vi "SEC code V4.1.vi"() -> ()   [LabVIEW 2020]
uses:
  SEC code V3.1/Drivers and Aux files/user.lib/atmcd32d.llb/Shutter_type typedef.ctl
  SEC code V3.1/Drivers and Aux files/State.ctl
  SEC code V3.1/Drivers and Aux files/SECenumctl.ctl
  SEC code V3.1/Drivers and Aux files/user.lib/atmcd32d.llb/TriggerMode_mode typedef.ctl
  SEC code V3.1/Drivers and Aux files/OSSPEC.ctl
  SEC code V3.1/Drivers and Aux files/OSPEC-enum.ctl
  Labview/IVIUM/IVIUM_remdriver.lvlib
panel:
  in  "Tab Control 5":enum32{"IVIUM", "iDUS", "Kymera"}(tab)
  out "current":dbl caption="Current (A)" format="%_4g"
  out "cell on":bool
  out "V (during measurment)":dbl
  out "Potentiostat Status":string
  out "T reached?":bool
  out "Shut down sequence run?":bool
  out "Curent Temp":i32
  in  "Tab Control 4":enum32{"SEC E", "SEC t", "Run"}(tab)
  in  "Start potential (V)":dbl=0.2
  in  "Stop potential (V)":dbl=0.7
  in  "Increment (V)":dbl=0.05
  in  "Default Potential (V)":dbl=0.2
  in  "Wait before \nspectrum (s)":dbl=0.1
  in  "Equilibration \ntime (s)":u32=5
  in  "Reverse Scan\ndirection":bool
  in  "(update and read)":bool
  in  "Tab Control 3":T1(tab)
  in  "Inetegration Time (us)":i32=5000
  in  "Continuous \nStrobe Delay (us)":i32
  in  "Use iDus?":bool=TRUE
  in  "Return detector \nto room T?":bool
  in  "Init, Cool, read dark,\nOR\nWarm/de-init detector":bool
  in  "Temperature\n(degrees C)":i32
  in  "Number of scans in kinetic cycle":i32=30
  in  "Exposure time (s)":dbl=0.03
  in  "Tab Control 2":T2(tab)
  in  "V 1 time (s)":dbl=10.0
  in  "V off time":dbl=30.0
  in  "Sampling time (s)":dbl
  in  "V 2 time (s)":dbl=20.0
  in  "Run OSPSEC":bool
  out "OCP":dbl format="%_3f"
  in  "V1 (V)":dbl=0.4
  in  "V2 (V)":dbl=0.8
  in  "Slow sample time (s)":dbl=1500.0
  out "Time during PD":u32
  in  "File Name":string="test-1"
  in  "Path":path=path "C:/Data"
  in  "Tab Control":T3(tab)
  out "?":T4(graph)
  out "?":cluster{i32[], dbl[]}(graph)
  out "?":T4(graph)
  out "?":T4(graph)
  out "?":cluster{dbl[], dbl[]}(graph)
  out "?":cluster{i32[], "array":i32[]}(graph)
  out "I_overload":bool
  out "Aninput1_overload":bool
  out "E_overload":bool
  out "cell-off button pressed":bool
  in  "Default\nCurrent range":T5(ring)=enum."100 uA"
  in  "Default Filter":T6(ring)=enum."10 kHz"
  out "Device serial number":string
  in  "Set Stability":T7(ring)=enum."Standard"
  out "Number of Spectrometers":i32
  out "IDus not in read loop? (kinetic)":bool
  out "Get status return code":dbl
  out "xpixels":i32
  out "ypixels":i32
  out "Calculated exposure time":sgl format="%.2f"
  out "Check timings return code":u32
  out "Set temprature\nreturn code":u32
  out "get aquired data return code":u32
  out "Start Aquisition return code":u32
  out "Init. return code":u32
  out "Cooler Off return code":u32
  out "Time before the start of current aquisition (ms)":u32
  out "Time  after the aquisition (before fetch data), (ms)":u32
  in  "Shutter opens on TTL":T8=enum."TTL High"
  in  "Shutter open and close time":i32
  out "Get aqisition ok? (kinetic mode)":bool
  out "Time taken to apply V2":u32
  out "Values to re-intialise to at end\nof the measument":T9
  out "ContinuousStrobe Out":u32
  out "Wrapper Out":u32
  out "WL Values":dbl[](array[numeric])
  in  "Exit and disconnect":bool
  # "Checklist for avoiding errors:\n(1) Light on the IVIUM should be blue with red flashes\nIf the system crahes and the light is red then connect and disconnect in IVUM soft/turn stat off/on\n(2) Maya Pro should read in ocean view/or the get intensity program\nIf maya is not reading connect and disconnect USB\n(3) If errors persist rrepeat steps 1 + 2 then re-compile code by clicking the\nwhite (run) whilst holding down CRTL + (left) SHIFT\n(4) At the end of a potential decay measurment click exit before starting a new measurment\n(5) IF USING THE iDus DO NOT EXIT WITHOUT WARMING CAMERA BACK TO ROOM T,YOU \nWILL DAMAGE IT"
  # "Program control"
  # "Potential decay control"
  # "Spectrometer control"
  # "System status"
  # "SEC control"
  # "Cell on?"
  # "Use the integration time program in the same folder as this program\nto get the optimum value. For kinetic mode the time resolution is limited \nby integration time"
  # "Unless you know what you are doing keep these at 0.03 and 30"
  # "I overload overload"
  # "off button pressed"
  # "Aninput1 overload"
  # "E overload"
  # "OSPEC loop exit"
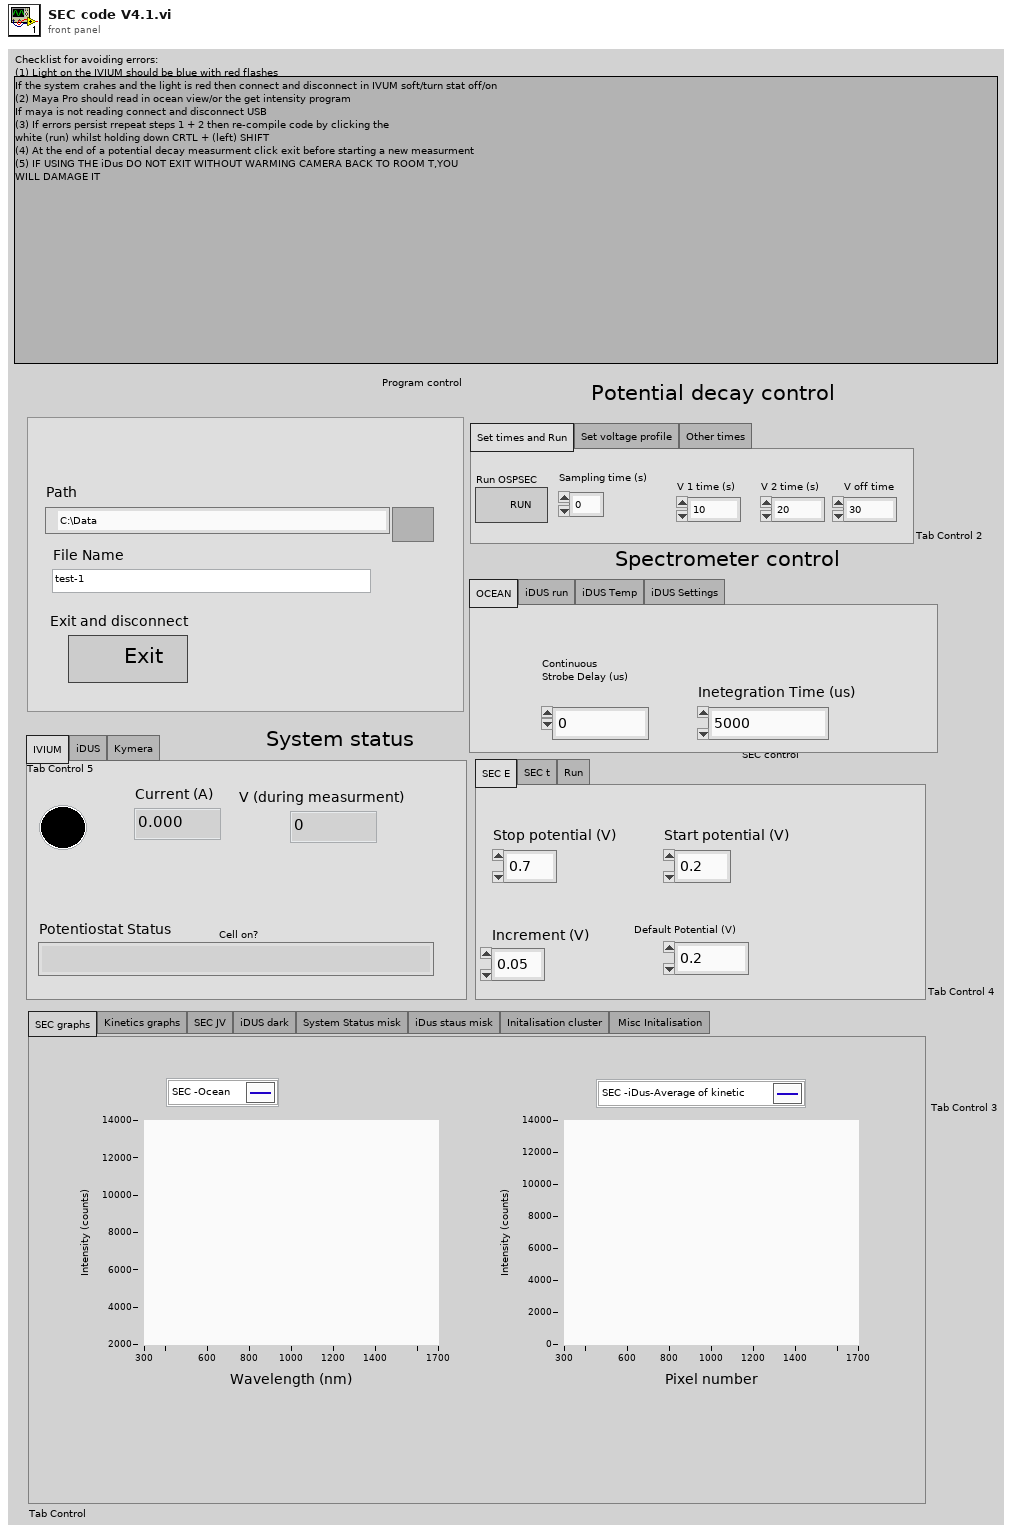
[diagram p1: front panel]
types:
  T1 = enum32{"OCEAN", "iDUS run", "iDUS Temp", "iDUS Settings"}
  T2 = enum32{"Set times and Run", "Set voltage profile", "Other times"}
  T3 = enum32{"SEC graphs", "Kinetics graphs", "SEC JV", "iDUS dark", "System Status misk", "iDus staus misk", "Initalisation cluster", "Misc Initalisation "}
  T4 = cluster{"WL Values":dbl[], "Spectrum Values":dbl[]}
  T5 = enum16{"10 A", "1 A", "100 mA", "10 mA", "1 mA", "100 uA", "10 uA", "1 uA", "100 nA", "10 nA", "1 nA", "100 pA", "10 pA", "1 pA"}
  T6 = enum16{"1 MHz", "100 kHz", "10 kHz", "1 kHz", "10 Hz"}
  T7 = enum16{"High Speed", "Standard", "High Stability"}
  T8 = typedef "Shutter_type typedef.ctl" = enum16{"TTL Low", "TTL High"}
  T9 = cluster{"Currents":dbl[], "Potentials":dbl[], "Device Status":string, "Device serial no":string, "Current":dbl, "Default \nPotential":dbl, "I overload":bool, "Cell On":bool, "E overload":bool, "Aninput1 overload":bool, "Cell off button pressed":bool, "Start potential":dbl, "Stop potential":dbl, "Increment":dbl, "SEC":dbl[], "Path":path, "File name":string}
  T10 = cluster{"Current array":dbl[], "Potential array":dbl[], "Status":string, "Serial No":string, "Current":dbl, "Default\n potential":dbl, "I overload":bool, "Cell on":bool, "E overload":bool, "Cell of button pressed":bool, "Aninput1 overload":bool, "Stop \npotential":dbl, "Start \npotential":dbl, "Increment":dbl, "Spectrum":dbl[][], "Path":path, "File Name":string, "Sample rate":dbl, "V2 time":dbl, "V off time":dbl, "V 2":dbl, "V 1":dbl, "V1 time":dbl, "Time array":dbl[], "Integration time":i32, "Continous strobe delay":i32, "Time elapsed ":i32, "Start time":i32, "Time for E measurment":i32[], "Time for I measurment ":i32[], "Time for spectrum measurment":i32[], "Return detector to \nroom T":bool, "Number of scans in kinetic cycle":i32, "Exposure time":i32}
  T11 = typedef "State.ctl" = enum16{"Initialize", "Wait for Event", "Run SEC", "Run OSPEC", "Initialse and cool iDus", "Exit"}
  T12 = typedef "SECenumctl.ctl" = enum16{"Read spectrum from Ocean", "Read spectrum from iDus", "Apply potential", "Wait"}
  T13 = typedef "TriggerMode_mode typedef.ctl" = enum16{"Internal", "External", "N/A (2)", "N/A (3)", "N/A (4)", "N/A (5)", "External Start", "External Exposure (Bulb)", "N/A (8)", "External FVB EM", "Software", "N/A (11)", "External Charge Shifting"}
  T14 = typedef "OSSPEC.ctl" = enum16{"Read Potential and spectrum", "Read current and spectrum", "Reinitialise Cell", "Apply V1", "End measurment", "Apply V2"}
  T15 = typedef "OSPEC-enum.ctl" = enum16{"Check exit", "Read", "Wait"}
  T16 = enum16{"off", "EStat4EL", "EStat2EL", "EStatDummy1", "EStatDummy2", "EStatDummy3", "EStatDummy4", "IStat4EL", "IStat2EL", "IStatDummy", "BiStat4EL", "BiStat2EL"}
  T17 = typedef "Error Code Enum typedef.ctl" = enum32{"N/A (0)", "DRV_ERROR_CODES", "DRV_SUCCESS", "DRV_VXDNOTINSTALLED", "DRV_ERROR_SCAN", "DRV_ERROR_CHECK_SUM", "DRV_ERROR_FILELOAD", "DRV_UNKNOWN_FUNC", "DRV_ERROR_VXD_INIT", "DRV_ERROR_ADDRESS", "DRV_ERROR_PAGELOCK", "DRV_ERROR_PAGEUNLOCK", "DRV_ERROR_BOARDTEST", "DRV_ERROR_ACK", "DRV_ERROR_UP_FIFO", "DRV_ERROR_PATTERN", "N/A (16)", "DRV_ACQUISITION_ERRORS", "DRV_ACQ_BUFFER", "DRV_ACQ_DOWNFIFO_FULL", "DRV_PROC_UNKONWN_INSTRUCTION", "DRV_ILLEGAL_OP_CODE", "DRV_KINETIC_TIME_NOT_MET", "DRV_ACCUM_TIME_NOT_MET", "DRV_NO_NEW_DATA", "N/A (25)", "DRV_SPOOLERROR", "N/A (27)", "N/A (28)", "N/A (29)", "N/A (30)", "N/A (31)", "N/A (32)", "DRV_TEMPERATURE_CODES", "DRV_TEMPERATURE_OFF", "DRV_TEMPERATURE_NOT_STABILIZED", "DRV_TEMPERATURE_STABILIZED", "DRV_TEMPERATURE_NOT_REACHED", "DRV_TEMPERATURE_OUT_RANGE", "DRV_TEMPERATURE_NOT_SUPPORTED", "DRV_TEMPERATURE_DRIFT", "N/A (41)", "N/A (42)", "N/A (43)", "N/A (44)", "N/A (45)", "N/A (46)", "N/A (47)", "N/A (48)", "DRV_GENERAL_ERRORS", "DRV_INVALID_AUX", "DRV_COF_NOTLOADED", "DRV_FPGAPROG", "DRV_FLEXERROR", "DRV_GPIBERROR", "N/A (55)", "N/A (56)", "N/A (57)", "N/A (58)", "N/A (59)", "N/A (60)", "N/A (61)", "N/A (62)", "N/A (63)", "DRV_DATATYPE", "DRV_DRIVER_ERRORS", "DRV_P1INVALID", "DRV_P2INVALID", "DRV_P3INVALID", "DRV_P4INVALID", "DRV_INIERROR", "DRV_COFERROR", "DRV_ACQUIRING", "DRV_IDLE", "DRV_TEMPCYCLE", "DRV_NOT_INITIALIZED", "DRV_P5INVALID", "DRV_P6INVALID", "DRV_INVALID_MODE", "DRV_INVALID_FILTER", "DRV_I2CERRORS", "DRV_I2CDEVNOTFOUND", "DRV_I2CTIMEOUT", "DRV_P7INVALID", "N/A (84)", "N/A (85)", "N/A (86)", "N/A (87)", "N/A (88)", "N/A (89)", "DRV_IOCERROR", "DRV_VRMVERSIONERROR"}
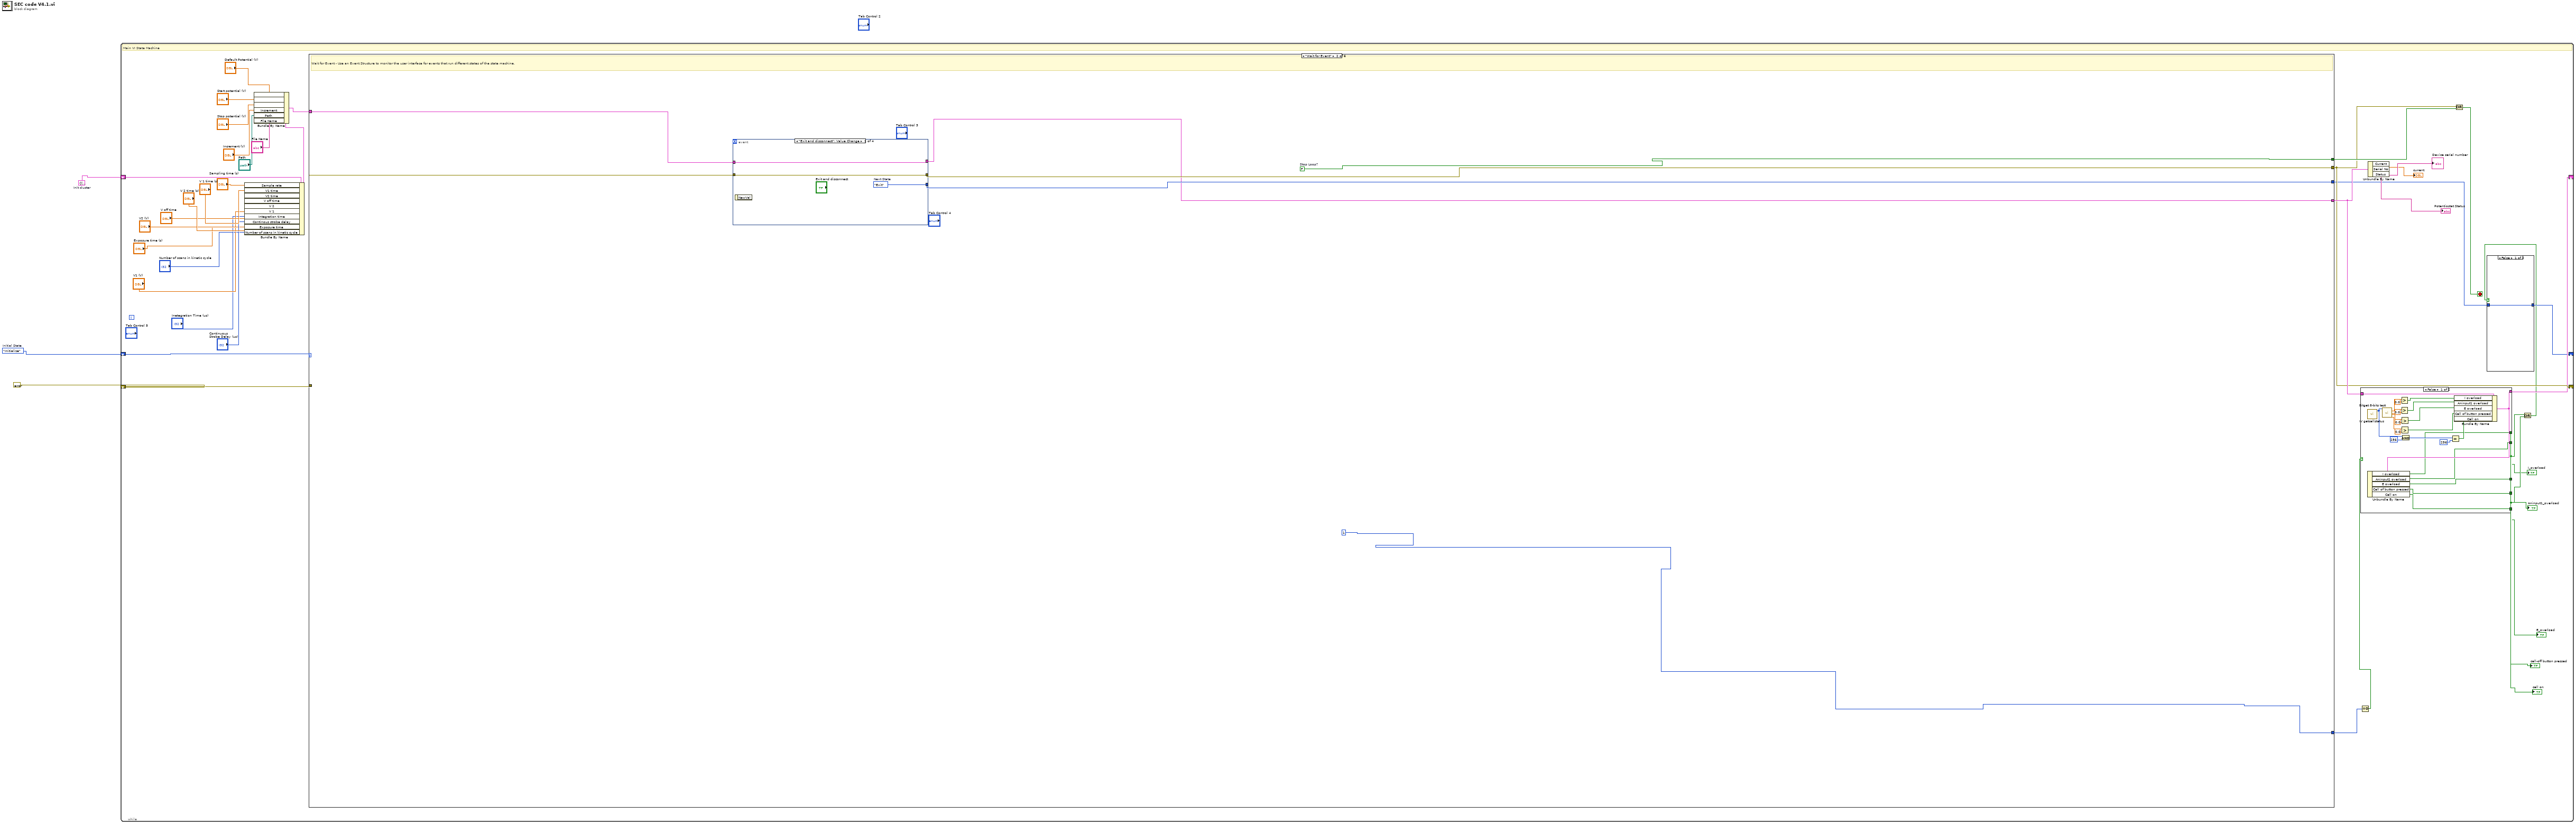
[diagram p0: block diagram]
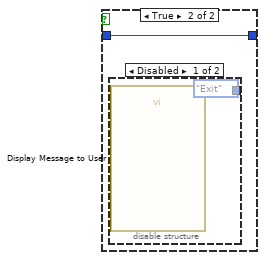
[diagram p2: hidden frame]
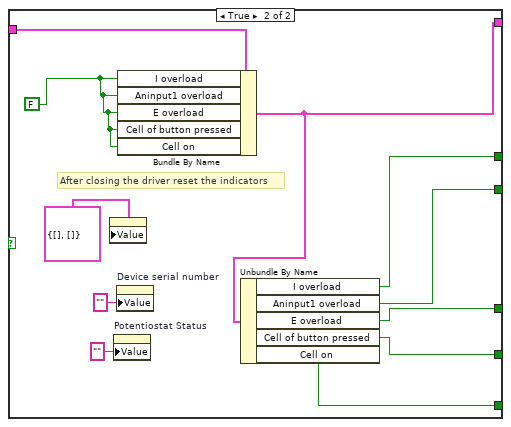
[diagram p4: hidden frame]
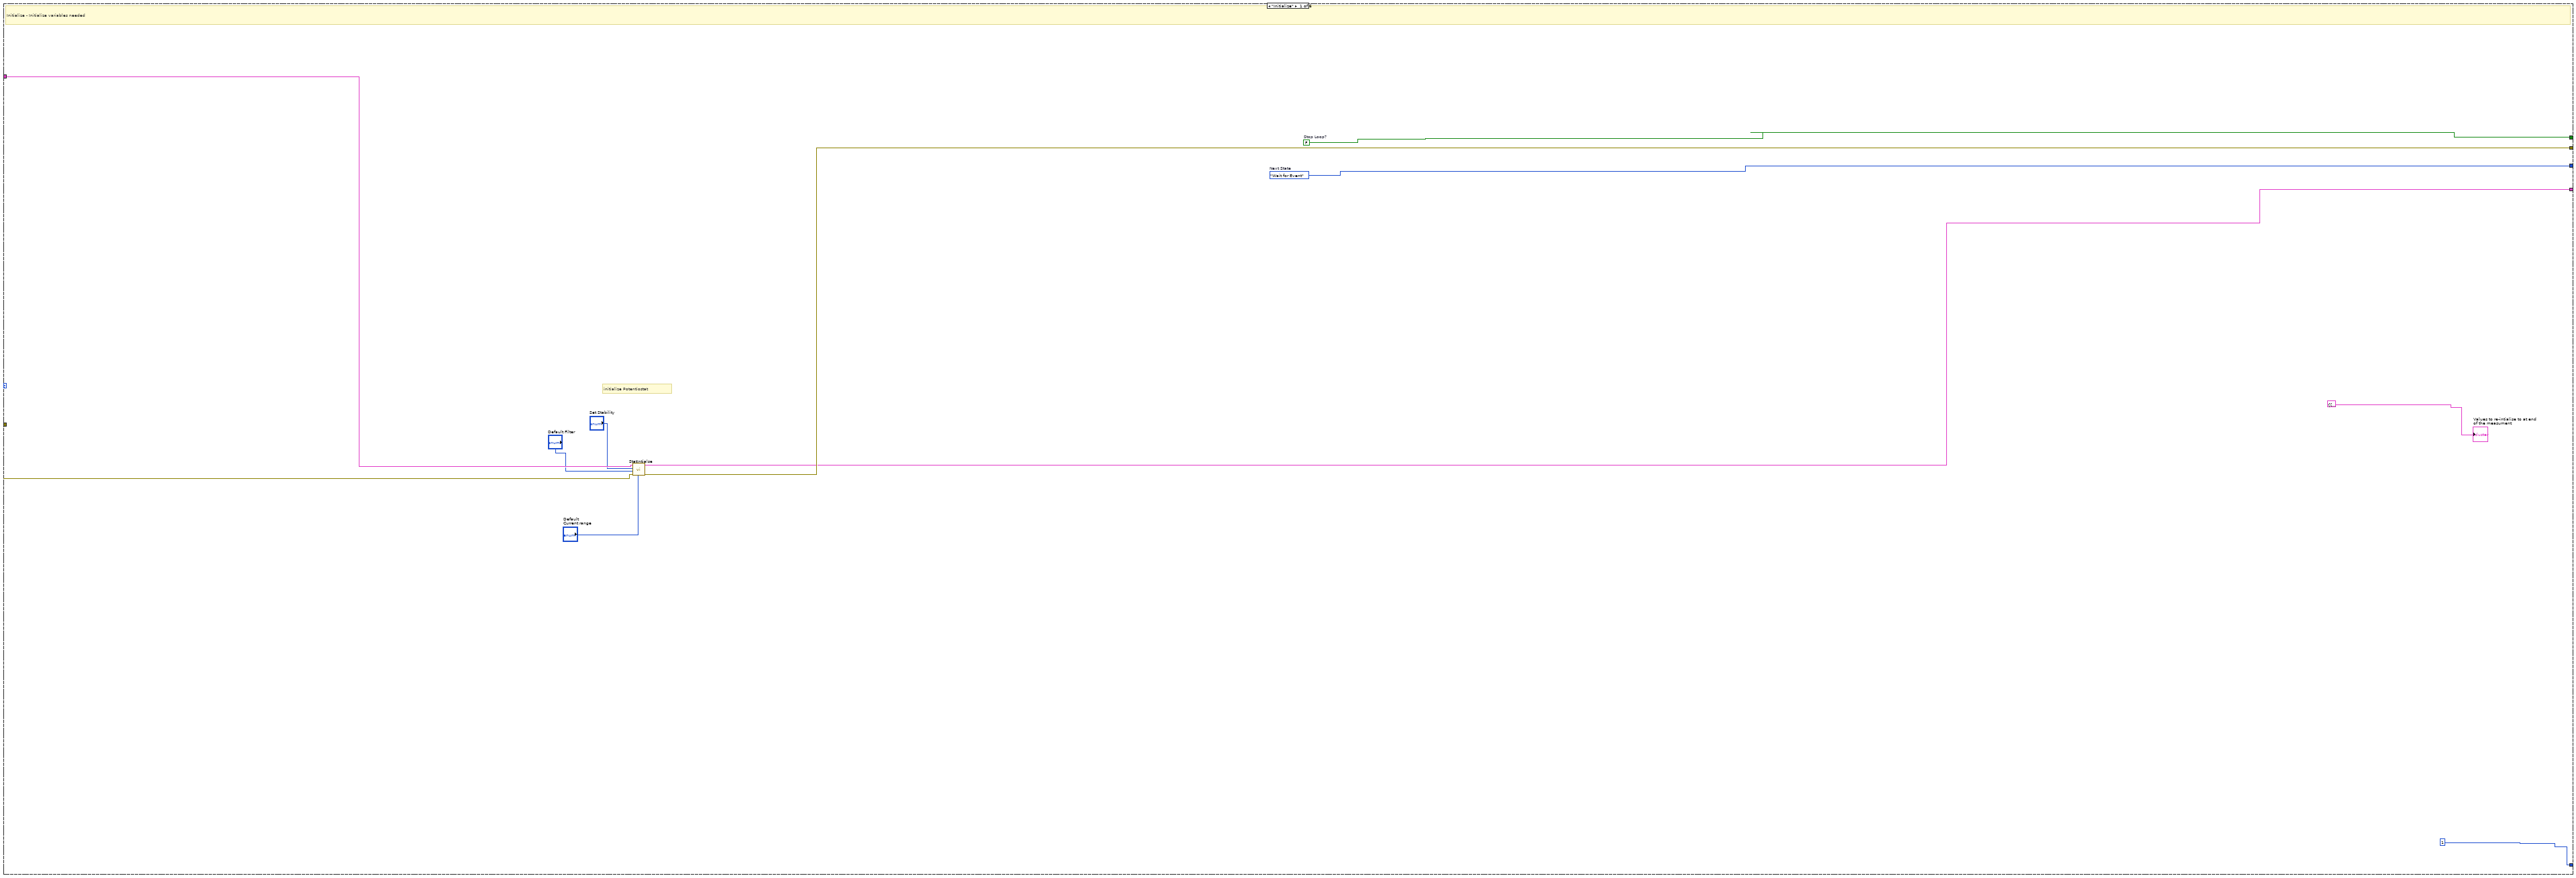
[diagram p5: hidden frame]
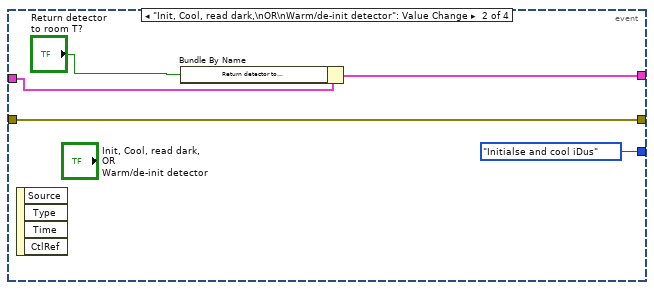
[diagram p6: hidden frame]
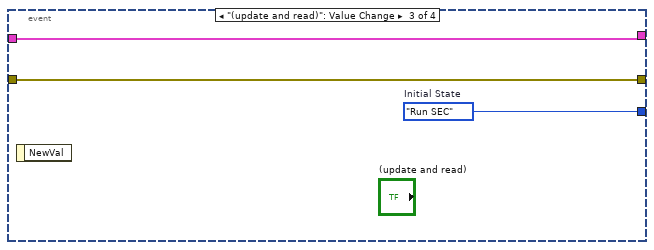
[diagram p7: hidden frame]
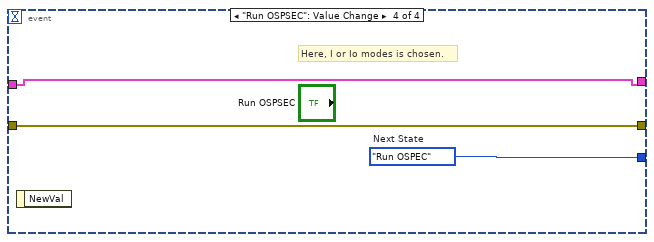
[diagram p8: hidden frame]
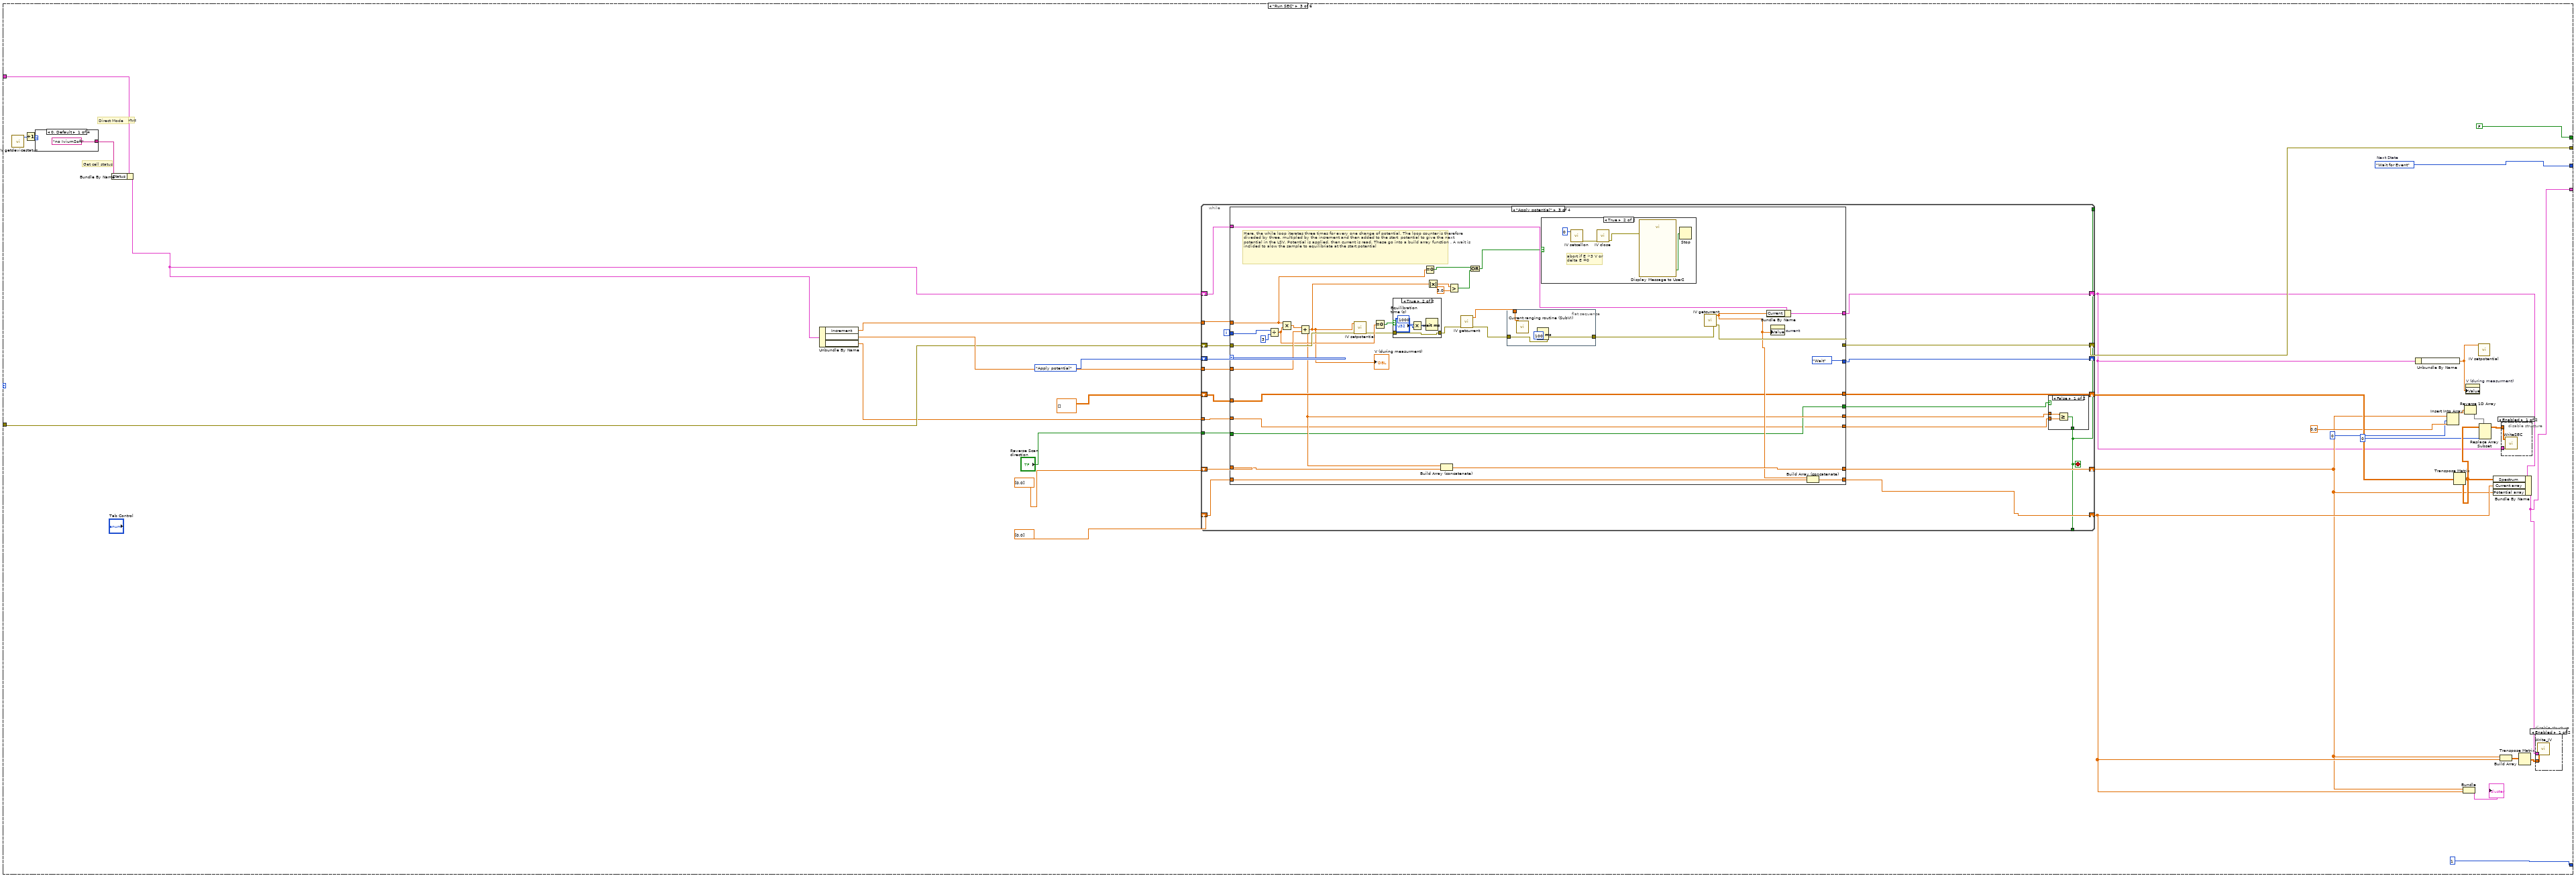
[diagram p9: hidden frame]
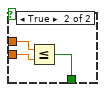
[diagram p12: hidden frame]
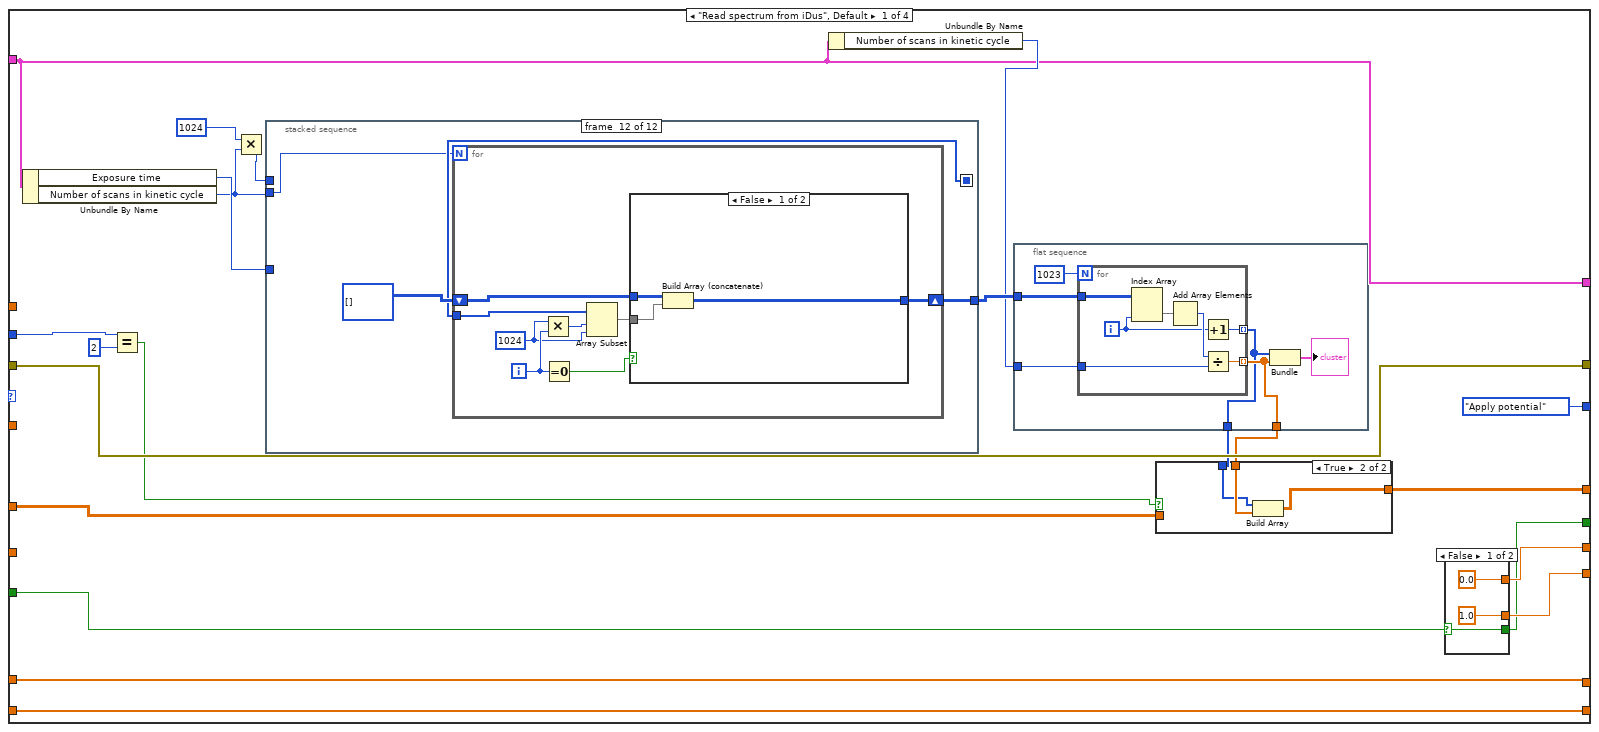
[diagram p13: hidden frame]
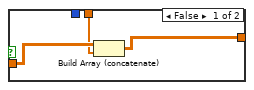
[diagram p14: hidden frame]
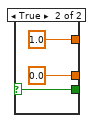
[diagram p15: hidden frame]
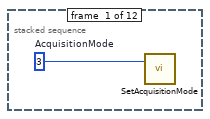
[diagram p16: hidden frame]
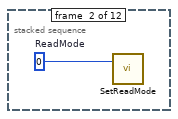
[diagram p17: hidden frame]
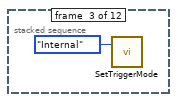
[diagram p18: hidden frame]
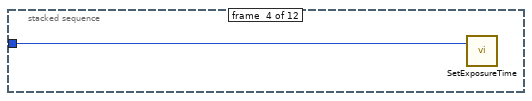
[diagram p19: hidden frame]
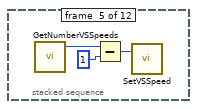
[diagram p20: hidden frame]
diagram:
  w1 = T10 {"Current array"=[], "Potential array"=[], "Status"="", "Serial No"="", "Current"=0.0, "Default\n potential"=0.0, "I overload"=FALSE, "Cell on"=FALSE, "E overload"=FALSE, "Cell of button pressed"=FALSE, "Aninput1 overload"=FALSE, "Stop \npotential"=0.0, "Start \npotential"=0.0, "Increment"=0.0, "Spectrum"=[], "Path"=path "", "File Name"="", "Sample rate"=0.0, "V2 time"=0.0, "V off time"=0.0, "V 2"=0.0, "V 1"=0.0, "V1 time"=0.0, "Time array"=[], "Integration time"=0, "Continous strobe delay"=0, "Time elapsed "=0, "Start time"=0, "Time for E measurment"=[], "Time for I measurment "=[], "Time for spectrum measurment"=[], "Return detector to \nroom T"=FALSE, "Number of scans in kinetic cycle"=0, "Exposure time"=0}  # Init cluster
  w3 = State."Initialize"  # Initial State
  n1 = while {
    shift-right: [w22] -> _
    shift-left: w3 -> [w42]
    shift-right: [w27] -> _
    shift-left: w1 -> [w17]
    shift-right: [w28] -> _
    shift-left: errorcluster {"status"=FALSE, "code"=0, "source"=""} ("error constant") -> [w41]
    stop <- w39 stop-if-true
    # "Main VI State Machine"
    n2 = Bundle By Name(cluster=w17, "Sample rate"="Sampling time (s)", "V1 time"="V 1 time (s)", "V2 time"="V 2 time (s)", "V off time"="V off time", "V 2"="V2 (V)", "V 1"="V1 (V)", "Integration time"="Inetegration Time (us)", "Continous strobe delay"="Continuous \nStrobe Delay (us)", "Exposure time"="Exposure time (s)", "Number of scans in kinetic cycle"="Number of scans in kinetic cycle") -> (w11:T10)
    n3 = Bundle By Name(cluster=w11, "Default\n potential"="Default Potential (V)", "Start \npotential"="Start potential (V)", "Stop \npotential"="Stop potential (V)", "Increment"="Increment (V)", "Path"="Path", "File Name"="File Name") -> (w24:T10)
    n4 = case shown="\"Wait for Event\"" w42 {
      tunnel: [w88 w98 w144 w368 State."Wait for Event" ("f") w1199] -> w7
      tunnel: [w87 w95 FALSE ("Stop Loop?") w367 FALSE ("Stop Loop?") _] -> w40
      tunnel: w24 -> [w85 w92 w131 w370 w390 w1197]
      tunnel: [w81 w93 w115 w370 w386 w1197] -> w35
      tunnel: w41 -> [w89 w97 w140 w373 w388 w1196]
      tunnel: [w90 w96 w139 w376 w387 w1196] -> w28
      tunnel: [1 ("devconnect") 1 ("devconnect") 1 ("devconnect") w371 1 ("devconnect") 1 ("devconnect")] -> w23
      frame "Initialize" {
        w87 = FALSE  # Stop Loop?
        w88 = State."Wait for Event"  # Next State
        # "initialize Potentiostat"
        # "Initialize - Initialize variables needed"
        n5 = call "StatIntialse.vi"("Init cluster 2"=w85, "Set Stability"="Set Stability", "Default\n Filter"="Default Filter", "error in (no error)"=w89, "Default\nCurrent range"="Default\nCurrent range") -> ("Init cluster"=w81:T10, "error out"=w90:errorcluster)  [unwired: 4 in]
        "Values to re-intialise to at end\nof the measument" <- T9 {"Currents"=[], "Potentials"=[], "Device Status"="", "Device serial no"="", "Current"=0.0, "Default \nPotential"=0.0, "I overload"=FALSE, "Cell On"=FALSE, "E overload"=FALSE, "Aninput1 overload"=FALSE, "Cell off button pressed"=FALSE, "Start potential"=0.0, "Stop potential"=0.0, "Increment"=0.0, "SEC"=[], "Path"=path "", "File name"=""} ("Values to re-intialise to at end\nof the measument")
      }
      frame "Wait for Event" {
        w95 = FALSE  # Stop Loop?
        # "Wait for Event - Use an Event Structure to monitor the user interface for events that run different states of the state machine."
        n6 = event shown="[0] \"Exit and disconnect\": Value Change" {
          selector: _ -> [_ _ _ _]
          dyn-events: _ -> [_ _ _ _]
          timeout: _ -> [_ _ _ _]
          tunnel: [w101 State."Initialse and cool iDus" ("Next State") w108 w112] -> w98
          tunnel: w97 -> [w100 w106 w109 w111]
          tunnel: [w100 w106 w109 w111] -> w96
          tunnel: w92 -> [w99 w104 w107 w110]
          tunnel: [w99 w102 w107 w110] -> w93
          event "Exit and disconnect": Value Change {
            w101 = State."Exit"  # Next State
            n7 = event-data() -> ()  [unwired: 1 in, 1 out]
          }
          event "Init, Cool, read dark,\nOR\nWarm/de-init detector": Value Change {
            n8 = event-data() -> ()  [unwired: 1 in, 4 out]
            n9 = Bundle By Name(cluster=w104, "Return detector to \nroom T"="Return detector \nto room T?") -> (w102:T10)
          }
          event "(update and read)": Value Change {
            w108 = State."Run SEC"  # Initial State
            n10 = event-data() -> ()  [unwired: 1 in, 1 out]
          }
          event "Run OSPSEC": Value Change {
            w112 = State."Run OSPEC"  # Next State
            # "Here, I or Io modes is chosen."
            n11 = event-data() -> ()  [unwired: 1 in, 1 out]
          }
        }
      }
      frame "Run SEC" {
        w144 = State."Wait for Event"  # Next State
        # "Get cell status"
        # "Get Device Status"
        # "Direct Mode"
        n12 = call "IV getdevicestatus.vi"() -> ("return type"=w143:i32)  [unwired: 10 in, 1 out]
        n13 = Increment(x=w143) -> (x+1=w142:i32)
        n14 = case shown="0, Default" w142 {
          tunnel: ["no IviumSoft" "device not connected" "device available_idle" "device available_busy"] -> w146
          frame 0, Default {
          }
          frame 1 {
          }
          frame 2 {
          }
          frame 3 {
          }
        }
        n15 = Bundle By Name(cluster=w131, "Status"=w146) -> (w117:T10)
        n16 = Unbundle By Name(w117) -> ("Increment"=w137:dbl, "Start \npotential"=w141:dbl, "Stop \npotential"=w132:dbl)
        n17 = while {
          shift-right: [w170] -> w114
          shift-left: w117 -> [w171]
          tunnel: w137 -> [w166]
          tunnel: w141 -> [w165]
          shift-right: [w167] -> w139
          shift-left: w140 -> [w168]
          shift-right: [w159] -> _
          shift-left: SECenumctl."Apply potential" -> [w163]
          shift-right: [w161] -> w116
          shift-left: dbl[] [0.0] -> [w160]
          shift-right: [w156] -> w120
          shift-left: dbl[] [0.0] -> [w157]
          tunnel: w132 -> [w158]
          shift-right: [w155] -> w130
          shift-left: dbl[][] [] -> [w154]
          tunnel: "Reverse Scan\ndirection" -> [w153]
          tunnel: [w151] -> _
          tunnel: [w151] -> _
          i -> [w169]
          stop <- w151 stop-if-true
          n18 = case shown="\"Apply potential\"" w163 {
            tunnel: w171 -> [w180 w280 w305 w335]
            tunnel: [w180 w280 w304 w335] -> w170
            tunnel: w169 -> [w187 _ w318 w344]
            tunnel: w168 -> [w189 w276 w315 w345]
            tunnel: [w189 w276 w306 w345] -> w167
            tunnel: w166 -> [_ _ w301 _]
            tunnel: w165 -> [_ _ w317 _]
            tunnel: [w193 w279 w298 w351] -> w164
            tunnel: [w192 w278 w290 w350] -> w162
            tunnel: [w194 w277 w309 w349] -> w161
            tunnel: w160 -> [w194 w277 w310 w349]
            tunnel: [SECenumctl."Apply potential" w281 SECenumctl."Wait" SECenumctl."Apply potential"] -> w159
            tunnel: w158 -> [_ _ w290 _]
            tunnel: w157 -> [w195 w272 w308 w346]
            tunnel: [w195 w272 w307 w346] -> w156
            tunnel: [w183 w271 w302 w338] -> w155
            tunnel: w154 -> [w184 w271 w302 w337]
            tunnel: w153 -> [w191 w270 w291 w336]
            tunnel: [w190 w269 w291 w336] -> w152
            frame "Read spectrum from iDus", Default {
              n19 = Unbundle By Name(w180) -> ("Exposure time"=w188:i32, "Number of scans in kinetic cycle"=w181:i32)
              n20 = Equal?(x=w187, y=2) -> (x = y?=w185:bool)
              n21 = Multiply(x=1024, y=w181) -> (x*y=w199:i32)
              n22 = stacked-sequence {
                seq-local: [_ _ _ _ _ _ _ _ _ _ w230 _] -> [_ _ _ _ _ _ _ _ _ _ _ w239]
                tunnel: [_ _ _ _ _ _ _ _ _ _ _ w240] -> w197
                tunnel: w181 -> [_ _ _ _ _ w219 _ _ _ _ _ w238]
                tunnel: w199 -> [_ _ _ _ _ _ _ _ _ _ w231 _]
                tunnel: w188 -> [_ _ _ w215 _ _ _ _ _ _ _ _]
                frame #0 {
                  w212 = u16 3  # AcquisitionMode
                  n23 = call "SetAcquisitionMode.vi"("mode"=w212) -> ()  [unwired: 1 in, 2 out]
                }
                frame #1 {
                  w213 = u16 0  # ReadMode
                  n24 = call "SetReadMode.vi"("mode"=w213) -> ()  [unwired: 1 in, 2 out]
                }
                frame #2 {
                  n25 = call "SetTriggerMode.vi"("mode"=TriggerMode_mode_typedef."Internal") -> ()  [unwired: 1 in, 2 out]
                }
                frame #3 {
                  n26 = call "SetExposureTime.vi"("time"=w215) -> ()  [unwired: 1 in, 2 out]
                }
                frame #4 {
                  n27 = call "GetNumberVSSpeeds.vi"() -> ("number"=w218:i32)  [unwired: 3 in, 2 out]
                  n28 = Subtract(x=w218, y=1) -> (x-y=w216:i32)
                  n29 = call "SetVSSpeed.vi"("index"=w216) -> ()  [unwired: 1 in, 2 out]
                }
                frame #5 {
                  n30 = call "SetNumberKinetics.vi"("number"=w219) -> ()  [unwired: 1 in, 2 out]
                }
                frame #6 {
                  w223 = 0  # Auto Shutter
                  n31 = call "SetShutter.vi"("type"=Shutter_type_typedef."TTL High", "mode"=w223, "closingtime"=0, "openingtime"=0) -> ()  [unwired: 10 in, 2 out]
                }
                frame #7 {
                  n32 = call "GetAcquisitionTimings.vi"() -> ("exposure"=w224:sgl)  [unwired: 11 in, 4 out]
                  n33 = property on="Calculated exposure time" class="DigNum (strict)"("Value"=w224) -> ()  [unwired: 2 in, 2 out]
                }
                frame #8 {
                  n34 = call "StartAcquisition.vi"() -> ("DLL error code"=w225:u32)  [unwired: 2 in, 1 out]
                  n35 = property on="Start Aquisition return code" class="DigNum (strict)"("Value"=w225) -> ()  [unwired: 2 in, 2 out]
                }
                frame #9 {
                  n36 = while {
                    stop <- w228 continue-if-true
                    w229 = u16 72  # DRV ACQUIRING
                    n37 = call "GetStatus.vi"() -> ("DLL error code"=→"Get status return code":u32, "status"=w227:T17)  [unwired: 3 in, 1 out]
                    n38 = Equal?(x=w227, y=w229) -> (x = y?=w228:bool)
                  }
                }
                frame #10 {
                  n39 = flat-sequence {
                    tunnel: [w233] -> w232
                    tunnel: w231 -> [w233]
                    tunnel: [w237] -> w230
                    tunnel: w232 -> [w235]
                    frame #0 {
                    }
                    frame #1 {
                      n40 = call "GetAcquiredData.vi"("size"=w235) -> ("DLL error code"=w234:u32, "array"=w237:i32[])  [unwired: 2 in, 1 out]
                      n41 = Equal?(x=20002 ("DRV_SUCCESS"), y=w234) -> ()  [unwired: 1 out]
                      n42 = property on="get aquired data return code" class="DigNum (strict)"("Value"=w234) -> ()  [unwired: 2 in, 2 out]
                    }
                  }
                }
                frame #11 {
                  n43 = for {
                    N: w238 -> [_]
                    shift-right: [w242] -> w240
                    shift-left: i32[][] [] -> [w244]
                    tunnel: w239 -> [w243]
                    i -> [w247]
                    w245 = 1024 ("x")
                    n44 = Multiply(x=w245, y=w247) -> (x*y=w249:i32)
                    n45 = Equal To 0?(x=w247) -> (x = 0?=w248:bool)
                    n46 = Array Subset(array=w243, index=w249, length=w245) -> (w246:i32[])
                    n47 = case shown="False" w248 {
                      tunnel: w246 -> [w251 w254]
                      tunnel: w244 -> [w252 _]
                      tunnel: [w250 w253] -> w242
                      frame False {
                        n48 = Build Array (concatenate)(w252, w251) -> (w250:i32[][])
                      }
                      frame True {
                        n49 = Build Array(w254) -> (w253:i32[][])
                      }
                    }
                  }
                }
              }
              n50 = Unbundle By Name(w180) -> ("Number of scans in kinetic cycle"=w182:i32)
              n51 = flat-sequence {
                tunnel: [w260] -> w178
                tunnel: w197 -> [w258]
                tunnel: w182 -> [w257]
                tunnel: [w255] -> w179
                frame #0 {
                  n52 = for {
                    N: 1023 -> [_]
                    tunnel: w258 -> [w265]
                    tunnel: [w266] -> w260 mode=indexing
                    tunnel: w257 -> [w263]
                    tunnel: [w261] -> w255 mode=indexing
                    i -> [w262]
                    n53 = Index Array(array=w265, index (col)=w262) -> (element=w264:i32[])  [unwired: 1 in]
                    n54 = Add Array Elements(numeric array=w264) -> (sum=w267:i32)
                    n55 = Increment(x=w262) -> (x+1=w261:i32)
                    n56 = Divide(x=w267, y=w263) -> (x/y=w266:dbl)
                  }
                  n57 = Bundle(w255, w260) -> (→"?":cluster{i32[], dbl[]})  [unwired: 1 in]
                }
              }
              n58 = case shown="True" w185 {
                tunnel: w184 -> [w202 _]
                tunnel: w178 -> [w201 w204]
                tunnel: [w200 w205] -> w183
                tunnel: w179 -> [_ w203]
                frame False {
                  n59 = Build Array (concatenate)(w202, w201) -> (w200:dbl[][])
                }
                frame True {
                  n60 = Build Array(w203, w204) -> (w205:dbl[][])
                }
              }
              n61 = case shown="False" w191 {
                selector: w191 -> [w206 w209]
                tunnel: [0.0 1.0] -> w193
                tunnel: [1.0 ("Stop \npotential") 0.0 ("Stop \npotential")] -> w192
                tunnel: [w206 w209] -> w190
                frame False {
                }
                frame True {
                }
              }
            }
            frame "Wait" {
              n62 = Multiply(x="Wait before \nspectrum (s)", y=1000.0) -> (x*y=w275:dbl)
              n63 = Wait (ms)(milliseconds to wait=w275) -> ()  [unwired: 1 out]
              n64 = case shown="False" "Use iDus?" {
                tunnel: [SECenumctl."Read spectrum from Ocean" SECenumctl."Read spectrum from iDus"] -> w281
                frame False {
                }
                frame True {
                }
              }
              n65 = case shown="False" w270 {
                selector: w270 -> [w284 w287]
                tunnel: [0.0 1.0] -> w279
                tunnel: [1.0 ("Stop \npotential") 0.0 ("Stop \npotential")] -> w278
                tunnel: [w284 w287] -> w269
                frame False {
                }
                frame True {
                }
              }
            }
            frame "Apply potential" {
              # "Here, the while loop iterates three times for every one change of potential. The loop counter is therefore diveded by three, multipled by the increment and then added to the start  potential to give the next potential in the LSV. Potential is applied, then current is read. These go into a build array function . A wait is inclided to alow the sample to equilibriate at the start potential"
              n66 = Divide(x=w318, y=3) -> (x/y=w313:dbl)
              n67 = Multiply(x=w301, y=w313) -> (x*y=w316:dbl)
              n68 = Add(x=w316, y=w317) -> (x+y=w298:dbl)
              "V (during measurment)" <- w298
              n69 = call "IV setpotential.vi"("error in (no error)"=w315, "value"=w298) -> ("error out"=w312:errorcluster)  [unwired: 7 in, 2 out]
              n70 = Equal To 0?(x=w313) -> (x = 0?=w314:bool)
              n71 = case shown="True" w314 {
                tunnel: w312 -> [w328 w330]
                tunnel: [w328 w330] -> w311
                frame False {
                }
                frame True {
                  n72 = Multiply(x=u32 1000, y="Equilibration \ntime (s)") -> (x*y=w329:u32)
                  n73 = Wait (ms)(milliseconds to wait=w329) -> ()  [unwired: 1 out]
                }
              }
              n74 = Equal To 0?(x=w301) -> (x = 0?=w296:bool)
              n75 = Absolute Value(x=w298) -> (abs(x)=w299:dbl)
              n76 = Build Array (concatenate)(w298, w310) -> (w309:dbl[])
              n77 = Greater?(x=w299, y=3.0) -> (0:w297:bool)
              n78 = call "IV getcurrent.vi"("error in (no error)"=w311) -> ("error out"=w294:errorcluster, "value out"=w292:dbl)  [unwired: 8 in, 1 out]
              n79 = Or(x=w296, y=w297) -> (x .or. y?=w295:bool)
              n80 = flat-sequence {
                tunnel: w294 -> [w322]
                tunnel: [w322] -> w293
                tunnel: w292 -> [w321]
                frame #0 {
                  n81 = call "Current ranging routine (SubVI).vi"("Current"=w321) -> ()  [unwired: 11 in]
                  n82 = Wait (ms)(milliseconds to wait=u32 100) -> ()  [unwired: 1 out]
                }
              }
              n83 = case shown="True" w295 {
                frame False {
                }
                frame True {
                  # "abort if E >3 V or\ndelta E =0"
                  n84 = call "IV setcellon.vi"("cellon"=0) -> ("error out"=w326:errorcluster)  [unwired: 8 in, 2 out]
                  n85 = call "IV close.vi"("error in (no error)"=w326) -> ("error out"=w324:errorcluster)  [unwired: 9 in, 1 out]
                  n86 = call "Display Message to User2"("error in (no error)"=w324) -> ("OK"=w327:bool)  [unwired: 9 in, 1 out]
                  n87 = Stop(stop? (T)=w327) -> ()
                }
              }
              n88 = call "IV getcurrent.vi"("error in (no error)"=w293) -> ("error out"=w306:errorcluster, "value out"=w303:dbl)  [unwired: 8 in, 1 out]
              n89 = Bundle By Name(cluster=w305, "Current"=w303) -> (w304:T10)
              n90 = property on="current" class="DigNum (strict)"("Value"=w303) -> ()  [unwired: 2 in, 2 out]
              n91 = Build Array (concatenate)(w303, w308) -> (w307:dbl[])
            }
            frame "Read spectrum from Ocean" {
              # "Building an matric of WL + intensities of multiple expts"
              n92 = Equal?(x=w344, y=2) -> (x = y?=w342:bool)
              n93 = Unbundle By Name(w335) -> ("Integration time"=w334:i32, "Continous strobe delay"=w333:i32)
              n94 = call "ReadSpectrum(SubVI).vi"("Continuous \nStrobe Delay"=w333, "Enter the \nInetegration Time"=w334) -> ("Spectrum Values"=w340:dbl[], "WL Values"=w341:dbl[], "Number of Spectrometers"=→"Number of Spectrometers":i32)  [unwired: 7 in]
              n95 = case shown="False" w342 {
                tunnel: w341 -> [_ w361]
                tunnel: w340 -> [w357 w360]
                tunnel: [w356 w359] -> w338
                tunnel: w337 -> [w358 _]
                frame False {
                  # "Matrix + int on i >3"
                  n96 = Build Array (concatenate)(w358, w357) -> (w356:dbl[][])
                }
                frame True {
                  # "WL + Int on =3"
                  n97 = Build Array(w361, w360) -> (w359:dbl[][])
                }
              }
              n98 = Bundle("WL Values"=w341, "Spectrum Values"=w340) -> (→"?":T4)  [unwired: 1 in]
              n99 = case shown="False" w336 {
                tunnel: [0.0 1.0] -> w351
                tunnel: [1.0 ("Stop \npotential") 0.0 ("Stop \npotential")] -> w350
                frame False {
                }
                frame True {
                }
              }
            }
          }
          n100 = case shown="False" w152 {
            tunnel: w164 -> [w174 w176]
            tunnel: w162 -> [w173 w175]
            tunnel: [w172 w177] -> w151
            frame False {
              n101 = Greater Or Equal?(x=w174, y=w173) -> (x >= y?=w172:bool)
            }
            frame True {
              n102 = Less Or Equal?(x=w176, y=w175) -> (x <= y?=w177:bool)
            }
          }
        }
        n103 = Unbundle By Name(w114) -> ("Default\n potential"=w136:dbl)
        n104 = Insert Into Array(array=w116, index=0, new element=0.0 ("new element/subarray")) -> (w126:dbl[])
        n105 = Transpose Matrix(1:w130) -> (0:w129:dbl[][])
        n106 = Bundle(w116, w120) -> (→"?":cluster{dbl[], dbl[]})  [unwired: 1 in]
        n107 = Reverse 1D Array(array=w126) -> (reversed array=w125:dbl[])
        n108 = property on="V (during measurment)" class="DigNum (strict)"("Value"=w136) -> ()  [unwired: 2 in, 2 out]
        n109 = call "IV setpotential.vi"("value"=w136) -> ()  [unwired: 8 in, 3 out]
        n110 = Replace Array Subset(array=w129, new element=w125, index (row)=0 ("index")) -> (w113:dbl[][])  [unwired: 1 in]
        n111 = Bundle By Name(cluster=w114, "Spectrum"=w129, "Current array"=w120, "Potential array"=w116) -> (w115:T10)
        n112 = Build Array(w116, w120) -> (w128:dbl[][])
        n113 = disable-structure shown="Enabled" {
          disable-tunnel: w113 -> [w150 _]
          disable-tunnel: w114 -> [w149 _]
          frame Enabled {
            n114 = call "WriteSEC.vi"("Init cluster"=w149, "Array"=w150) -> ()  [unwired: 10 in]
          }
          frame Disabled {
          }
        }
        n115 = Transpose Matrix(1:w128) -> (0:w127:dbl[][])
        n116 = disable-structure shown="Enabled" {
          disable-tunnel: w127 -> [w148 _]
          disable-tunnel: w115 -> [w147 _]
          frame Enabled {
            n117 = call "Write_JV.vi"("Init cluster"=w147, "Array"=w148) -> ()  [unwired: 10 in]
          }
          frame Disabled {
          }
        }
      }
      frame "Exit" {
        w366 = FALSE ("Shut down sequence run?")
        w367 = TRUE  # Stop Loop?
        w368 = State."Exit"  # (Value Not Used)
        # "This re-initialises a display for the iDus camera"
        # "On"
        # "Switch cell on/off"
        # "Diconnect device and close Ivium remdriver"
        # "Disconnect Ivium device (when connected)\nbefore terminating this VI"
        # "Close Ivium Driver"
        # "Exit - Exit the application."
        n118 = To Long Integer(number=0) -> (32bit integer=w375:i32)
        n119 = call "IV setcellon.vi"("error in (no error)"=w373, "cellon"=w375) -> ("error out"=w372:errorcluster)  [unwired: 7 in, 2 out]
        n120 = call "IV getdevicestatus.vi"("error in (no error)"=w372) -> ("error out"=w377:errorcluster, "return type"=w378:i32)  [unwired: 9 in]
        n121 = Greater Than 0?(x=w378) -> (x > 0?=w369:bool)
        n122 = case shown="True" w369 {
          tunnel: [w381 w383] -> w379
          tunnel: w377 -> [w381 _]
          tunnel: [0 ("devconnect") w382] -> w371
          frame False {
          }
          frame True {
            w382 = 0 ("devconnect")
            n123 = call "IV connect.vi"("devconnect"=w382) -> ("error out"=w383:errorcluster)  [unwired: 8 in, 2 out]
          }
        }
        n124 = property on="Shut down sequence run?" class="Bool (strict)"("Value"=w366) -> ()  [unwired: 2 in, 2 out]
        n125 = property on="Return detector \nto room T?" class="Bool (strict)"("Value"=w366) -> ()  [unwired: 2 in, 2 out]
        n126 = call "IV close.vi"("error in (no error)"=w379) -> ("error out"=w376:errorcluster)  [unwired: 9 in, 1 out]
      }
      frame "Run OSPEC" {
        # "Get cell status"
        # "Get Device Status"
        # "Direct Mode"
        n127 = call "IV getdevicestatus.vi"() -> ("return type"=w393:i32)  [unwired: 10 in, 1 out]
        n128 = Increment(x=w393) -> (x+1=w392:i32)
        n129 = case shown="0, Default" w392 {
          tunnel: ["no IviumSoft" "device not connected" "device available_idle" "device available_busy"] -> w391
          frame 0, Default {
          }
          frame 1 {
          }
          frame 2 {
          }
          frame 3 {
          }
        }
        n130 = Bundle By Name(cluster=w390, "Status"=w391) -> (w389:T10)
        n131 = while {
          shift-right: [w396] -> w387
          shift-left: w388 -> [w401]
          shift-right: [w397] -> w386
          shift-left: w389 -> [w403]
          shift-right: [w400] -> _
          shift-left: OSSPEC."Apply V1" -> [w402]
          i -> [w399]
          stop <- w398 stop-if-true
          n132 = case shown="\"Read Potential and spectrum\", Default" w402 {
            tunnel: w403 -> [w404 w689 w1059 w1082 w1119 w1153]
            tunnel: w401 -> [w407 w692 w1063 w1077 w1122 w1180]
            tunnel: [OSSPEC."End measurment" w709 OSSPEC."Read Potential and spectrum" OSSPEC."Read current and spectrum" OSSPEC."Read current and spectrum" OSSPEC."End measurment"] -> w400
            tunnel: [w413 w691 w1062 w1072 w1123 w1175] -> w396
            tunnel: [w414 w700 w1059 w1074 w1119 w1153] -> w397
            tunnel: w399 -> [_ _ _ _ _ _]
            tunnel: [FALSE FALSE FALSE FALSE FALSE TRUE] -> w398
            frame "Read Potential and spectrum", Default {
              n133 = flat-sequence {
                tunnel: w407 -> [w629]
                tunnel: [w628] -> w409
                tunnel: w409 -> [w632]
                tunnel: [w631] -> w408
                tunnel: [w633] -> w406
                tunnel: w408 -> [w633]
                frame #0 {
                  n134 = To Long Integer(number=T16."IStat4EL" ("Configuration")) -> (32bit integer=w627:i32)
                  n135 = call "IV setconnectionmode.vi"("error in (no error)"=w629, "value"=w627) -> ("error out"=w628:errorcluster)  [unwired: 7 in, 2 out]
                }
                frame #1 {
                  n136 = call "IV setcurrent.vi"("error in (no error)"=w632, "value"=0.0) -> ("error out"=w631:errorcluster)  [unwired: 7 in, 2 out]
                }
                frame #2 {
                }
              }
              n137 = Unbundle By Name(w404) -> ("Spectrum"=w416:dbl[][])
              n138 = Unbundle By Name(w404) -> ("Time for spectrum measurment"=w415:i32[], "Start time"=w418:i32)
              n139 = Unbundle By Name(w404) -> ("Potential array"=w411:dbl[])
              n140 = property on="Use iDus?" class="Bool (strict)"() -> ("Value"=w405:bool)  [unwired: 2 in, 2 out]
              n141 = Unbundle By Name(w404) -> ("Time for E measurment"=w410:i32[], "Start time"=w417:i32)
              n142 = case shown="True" w405 {
                tunnel: [w438 w501] -> w423
                tunnel: [w437 w502] -> w422
                tunnel: w418 -> [w436 w508]
                tunnel: w416 -> [w435 w506]
                tunnel: w415 -> [w433 w504]
                tunnel: [w432 w503] -> w412
                tunnel: w404 -> [w431 w507]
                frame False {
                  n143 = local read "Wrapper Out"() -> (w429:u32)
                  n144 = local read "ContinuousStrobe Out"() -> (w430:u32)
                  n145 = local read "WL Values"() -> (w428:dbl[])
                  n146 = while {
                    shift-right: [w454] -> _
                    shift-left: w431 -> [w455]
                    shift-right: [w447] -> _
                    shift-left: OSPEC-enum."Read" -> [w456]
                    shift-right: [w452] -> w437
                    shift-left: w433 -> [w451]
                    shift-right: [w446] -> w432
                    shift-left: w435 -> [w450]
                    shift-right: [w449] -> w438
                    shift-left: w436 -> [w440]
                    tunnel: w429 -> [w445]
                    tunnel: [w444] -> w434
                    tunnel: w430 -> [w443]
                    tunnel: w428 -> [w442]
                    tunnel: [w441] -> w427
                    i -> [w448]
                    stop <- w453 stop-if-true
                    n147 = case shown="\"Check exit\"" w456 {
                      tunnel: w455 -> [w465 w471 w495]
                      tunnel: [w465 w471 w495] -> w454
                      tunnel: [w463 FALSE FALSE] -> w453
                      tunnel: [w467 w483 w493] -> w452
                      tunnel: w451 -> [w467 w482 w493]
                      tunnel: w448 -> [_ _ _]
                      tunnel: [w462 w477 w489] -> w446
                      tunnel: w450 -> [w462 w481 w489]
                      tunnel: [w464 w468 w486] -> w449
                      tunnel: w440 -> [w464 _ w486]
                      tunnel: [OSPEC-enum."Wait" OSPEC-enum."Check exit" OSPEC-enum."Read"] -> w447
                      tunnel: w445 -> [w460 w475 w490]
                      tunnel: [w461 w476 w491] -> w444
                      tunnel: w443 -> [w461 w476 w491]
                      tunnel: w442 -> [_ w474 _]
                      tunnel: [w460 w475 w490] -> w441
                      frame "Check exit" {
                        n148 = Unbundle By Name(w465) -> ("V off time"=w459:dbl)
                        n149 = Multiply(x=w459, y=1000.0) -> (x*y=w457:dbl)
                        n150 = Greater Or Equal?(x=w464, y=w457) -> (x >= y?=w463:bool)
                      }
                      frame "Read", Default {
                        # "Continue 2d matrix of specta"
                        # "Continue to add times to this"
                        n151 = call "Wrapper_getSpectrum.vi"("Index"=0, "Wrapper"=w475) -> ("Spectrum Values"=w473:dbl[])  [unwired: 1 out]
                        n152 = Tick Count (ms)() -> (millisecond timer value=w469:u32)
                        n153 = Unbundle By Name(w471) -> ("Start time"=w470:i32)
                        n154 = Subtract(x=w469, y=w470) -> (x-y=w468:u32)
                        "Time during PD" <- w468
                        n155 = Bundle("WL Values"=w474, "Spectrum Values"=w473) -> (→"?":T4)  [unwired: 1 in]
                        n156 = Build Array (concatenate)(w482, w468) -> (w483:u32[])
                        n157 = Build Array (concatenate)(w481, w473) -> (w477:dbl[][])
                      }
                      frame "Wait" {
                        n158 = Unbundle By Name(w495) -> ("Sample rate"=w496:dbl)
                        n159 = Multiply(x=1000.0, y="Slow sample time (s)") -> (x*y=w485:dbl)
                        n160 = Greater?(x=w486, y=w485) -> (0:w484:bool)
                        n161 = case shown="True" w484 {
                          tunnel: w496 -> [w497 _]
                          frame False {
                            n162 = Multiply(x=w497, y=1000.0) -> (x*y=w499:dbl)
                            n163 = Wait (ms)(milliseconds to wait=w499) -> ()  [unwired: 1 out]
                          }
                          frame True {
                            # "slow down read to measure slow decays\nwithout oversampling"
                            n164 = Wait (ms)(milliseconds to wait=u32 500) -> ()  [unwired: 1 out]
                          }
                        }
                      }
                    }
                  }
                  n165 = call "End spectrum measurment.vi"("ContinuousStrobe Out"=w434, "Wrapper Out"=w427) -> ()  [unwired: 10 in]
                }
                frame True {
                  n166 = while {
                    shift-right: [w518] -> w501
                    shift-left: w508 -> [w519]
                    shift-right: [w511] -> _
                    shift-left: OSPEC-enum."Wait" -> [w520]
                    shift-right: [w517] -> w502
                    shift-left: w504 -> [w516]
                    shift-right: [w510] -> w503
                    shift-left: w506 -> [w515]
                    shift-right: [w514] -> _
                    shift-left: w507 -> [w513]
                    i -> [w512]
                    stop <- w509 stop-if-true
                    n167 = case shown="\"Read\", Default" w520 {
                      tunnel: w519 -> [w522 _ w623]
                      tunnel: [w522 w531 w623] -> w518
                      tunnel: [w528 FALSE FALSE] -> w509
                      tunnel: [w530 w535 w621] -> w517
                      tunnel: w516 -> [w530 w539 w621]
                      tunnel: w512 -> [_ w542 _]
                      tunnel: w515 -> [w523 w538 w617]
                      tunnel: [w529 w533 w619] -> w514
                      tunnel: w513 -> [w529 w533 w619]
                      tunnel: [OSPEC-enum."Wait" OSPEC-enum."Check exit" OSPEC-enum."Read"] -> w511
                      tunnel: [w523 w536 w617] -> w510
                      frame "Check exit" {
                        n168 = Unbundle By Name(w529) -> ("V off time"=w524:dbl)
                        n169 = Multiply(x=w524, y=1000.0) -> (x*y=w525:dbl)
                        n170 = Greater Or Equal?(x=w522, y=w525) -> (x >= y?=w528:bool)
                      }
                      frame "Read", Default {
                        n171 = Unbundle By Name(w533) -> ("Start time"=w532:i32)
                        n172 = property on="Number of scans in kinetic cycle" class="DigNum (strict)"() -> ("Value"=w534:i32)  [unwired: 2 in, 2 out]
                        n173 = Tick Count (ms)() -> (millisecond timer value=w540:u32)
                        n174 = call "GetDetector.vi"() -> ("xpixels"=w541:i32)  [unwired: 4 in, 3 out]
                        n175 = Subtract(x=w540, y=w532) -> (x-y=w531:u32)
                        n176 = Equal?(x=w542, y=1.0) -> (x = y?=w537:bool)
                        n177 = stacked-sequence {
                          seq-local: [_ _ _ _ _ _ _ _ _ _ w576 _] -> [_ _ _ _ _ _ _ _ _ _ _ w596]
                          seq-local: [_ _ _ _ _ _ _ _ w561 _ _ _] -> [_ _ _ _ _ _ _ _ _ _ _ w594]
                          seq-local: [_ _ _ _ _ _ _ _ _ _ w575 _] -> [_ _ _ _ _ _ _ _ _ _ _ w595]
                          tunnel: [_ _ _ _ _ _ _ _ _ _ _ w589] -> w536
                          tunnel: [_ _ _ _ _ _ _ _ _ _ _ w590] -> w535
                          tunnel: w534 -> [_ _ _ _ _ w554 _ _ _ _ _ w588]
                          tunnel: w531 -> [_ _ _ _ _ _ _ _ _ _ _ w591]
                          tunnel: w531 -> [_ _ _ _ _ _ _ _ _ _ _ _]
                          tunnel: w541 -> [_ w547 _ _ _ _ _ _ _ _ _ _]
                          tunnel: w532 -> [_ _ _ _ _ _ _ _ w560 _ w574 _]
                          tunnel: w539 -> [_ _ _ _ _ _ _ _ _ _ _ w587]
                          tunnel: w538 -> [_ _ _ _ _ _ _ _ _ _ _ w586]
                          tunnel: w537 -> [_ _ _ _ _ _ _ _ _ _ _ w585]
                          frame #0 {
                            w546 = u16 3  # AcquisitionMode
                            n178 = call "SetAcquisitionMode.vi"("mode"=w546) -> ()  [unwired: 1 in, 2 out]
                          }
                          frame #1 {
                            w548 = u16 0  # ReadMode
                            n179 = property on="xpixels" class="DigNum (strict)"("Value"=w547) -> ()  [unwired: 2 in, 2 out]
                            n180 = call "SetReadMode.vi"("mode"=w548) -> ()  [unwired: 1 in, 2 out]
                          }
                          frame #2 {
                            n181 = call "SetTriggerMode.vi"("mode"=TriggerMode_mode_typedef."Internal") -> ()  [unwired: 1 in, 2 out]
                          }
                          frame #3 {
                            n182 = property on="Exposure time (s)" class="DigNum (strict)"() -> ("Value"=w550:dbl)  [unwired: 2 in, 2 out]
                            n183 = call "SetExposureTime.vi"("time"=w550) -> ()  [unwired: 1 in, 2 out]
                          }
                          frame #4 {
                            n184 = call "GetNumberVSSpeeds.vi"() -> ("number"=w553:i32)  [unwired: 3 in, 2 out]
                            n185 = Subtract(x=w553, y=1) -> (x-y=w551:i32)
                            n186 = call "SetVSSpeed.vi"("index"=w551) -> ()  [unwired: 1 in, 2 out]
                          }
                          frame #5 {
                            n187 = call "SetNumberKinetics.vi"("number"=w554) -> ()  [unwired: 1 in, 2 out]
                          }
                          frame #6 {
                            w557 = 0  # Auto Shutter
                            n188 = property on="Shutter open and close time" class="DigNum (strict)"() -> ("Value"=w555:i32)  [unwired: 2 in, 2 out]
                            n189 = property on="Shutter opens on TTL" class="Enum (strict)"() -> ("Value"=w556:T8)  [unwired: 2 in, 2 out]
                            n190 = call "SetShutter.vi"("type"=w556, "mode"=w557, "closingtime"=w555, "openingtime"=w555) -> ()  [unwired: 10 in, 2 out]
                          }
                          frame #7 {
                            # "Meybe delete the exposure time insupt here"
                            n191 = property on="Exposure time (s)" class="DigNum (strict)"() -> ("Value"=w559:dbl)  [unwired: 2 in, 2 out]
                            n192 = call "GetAcquisitionTimings.vi"("exposure input"=w559) -> ("exposure"=w558:sgl)  [unwired: 10 in, 4 out]
                            n193 = property on="Calculated exposure time" class="DigNum (strict)"("Value"=w558) -> ()  [unwired: 2 in, 2 out]
                          }
                          frame #8 {
                            n194 = flat-sequence {
                              tunnel: [w562] -> w561
                              tunnel: w560 -> [w563]
                              frame #0 {
                                n195 = Tick Count (ms)() -> (millisecond timer value=w564:u32)
                                n196 = Subtract(x=w564, y=w563) -> (x-y=w562:u32)
                                n197 = property on="Time before the start of current aquisition (ms)" class="DigNum (strict)"("Value"=w562) -> ()  [unwired: 2 in, 2 out]
                              }
                              frame #1 {
                                n198 = call "StartAcquisition.vi"() -> ("DLL error code"=w565:u32)  [unwired: 2 in, 1 out]
                                n199 = property on="Start Aquisition return code" class="DigNum (strict)"("Value"=w565) -> ()  [unwired: 2 in, 2 out]
                              }
                            }
                          }
                          frame #9 {
                            n200 = while {
                              stop <- w569 continue-if-true
                              w570 = u16 72  # DRV ACQUIRING
                              n201 = call "GetStatus.vi"() -> ("DLL error code"=w567:u32, "status"=w568:T17)  [unwired: 3 in, 1 out]
                              n202 = property on="Get status return code" class="DigNum (strict)"("Value"=w567) -> ()  [unwired: 2 in, 2 out]
                              n203 = Equal?(x=w568, y=w570) -> (x = y?=w569:bool)
                              n204 = property on="IDus not in read loop? (kinetic)" class="Bool (strict)"("Value"=FALSE ("IDus not in read loop? (kinetic)")) -> ()  [unwired: 2 in, 2 out]
                            }
                          }
                          frame #10 {
                            n205 = flat-sequence {
                              tunnel: [w577] -> w575
                              tunnel: w574 -> [w578]
                              tunnel: [w584] -> w576
                              tunnel: w573 -> [w581]
                              frame #0 {
                                n206 = Tick Count (ms)() -> (millisecond timer value=w579:u32)
                                n207 = Subtract(x=w579, y=w578) -> (x-y=w577:u32)
                                n208 = property on="Time  after the aquisition (before fetch data), (ms)" class="DigNum (strict)"("Value"=w577) -> ()  [unwired: 2 in, 2 out]
                              }
                              frame #1 {
                                n209 = call "GetAcquiredData.vi"("size"=w581) -> ("DLL error code"=w582:u32, "array"=w584:i32[])  [unwired: 2 in, 1 out]
                                n210 = Equal?(x=20002 ("DRV_SUCCESS"), y=w582) -> (x = y?=w580:bool)
                                n211 = property on="get aquired data return code" class="DigNum (strict)"("Value"=w582) -> ()  [unwired: 2 in, 2 out]
                                n212 = property on="Get aqisition ok? (kinetic mode)" class="Bool (strict)"("Value"=w580) -> ()  [unwired: 2 in, 2 out]
                              }
                            }
                            n213 = property on="Number of scans in kinetic cycle" class="DigNum (strict)"() -> ("Value"=w571:i32)  [unwired: 2 in, 2 out]
                            n214 = Multiply(x=1024.0, y=w571) -> (x*y=w573:dbl)
                          }
                          frame #11 {
                            n215 = Subtract(x=w595, y=w594) -> (x-y=w593:u32)
                            n216 = Divide(x=w593, y=w588) -> (x/y=w592:dbl)
                            n217 = for {
                              N: w588 -> [_]
                              tunnel: w596 -> [w610]
                              tunnel: w592 -> [w608]
                              tunnel: w591 -> [w606]
                              shift-right: [w604] -> w589
                              shift-left: w586 -> [w603]
                              shift-right: [w600] -> w590
                              shift-left: w587 -> [w601]
                              tunnel: w585 -> [_]
                              i -> [w598]
                              w605 = 1024 ("x")
                              n218 = Multiply(x=w598, y=w608) -> (x*y=w607:dbl)
                              n219 = Multiply(x=w605, y=w598) -> (x*y=w609:i32)
                              n220 = Add(x=w607, y=w606) -> (x+y=w602:dbl)
                              n221 = Array Subset(array=w610, index=w609, length=w605) -> (w597:i32[])
                              n222 = Equal To 0?(x=w598) -> (x = 0?=w599:bool)
                              n223 = case shown="True" w599 {
                                tunnel: w597 -> [_ w612]
                                frame False {
                                }
                                frame True {
                                n224 = for {
                                N: 1023 -> [_]
                                tunnel: [w615] -> w613 mode=indexing
                                i -> [w616]
                                n225 = Increment(x=w616) -> (x+1=w615:i32)
                                }
                                n226 = Bundle(w613, w612) -> (w611:cluster{i32[], i32[]})  [unwired: 1 in]
                                n227 = property class="XYGraph (strict)"("Value"=w611) -> ()  [unwired: 2 in, 2 out]
                                }
                              }
                              n228 = Build Array (concatenate)(w603, w597) -> (w604:dbl[][])
                              n229 = Build Array (concatenate)(w601, w602) -> (w600:dbl[])
                            }
                          }
                        }
                      }
                      frame "Wait" {
                        n230 = Unbundle By Name(w619) -> ("Sample rate"=w618:dbl)
                        n231 = Multiply(x=w618, y=1000.0) -> (x*y=w625:dbl)
                        n232 = Wait (ms)(milliseconds to wait=w625) -> ()  [unwired: 1 out]
                      }
                    }
                    n233 = case shown="True" w509 {
                      selector: w509 -> [_ w521]
                      frame False {
                      }
                      frame True {
                        n234 = property on="IDus not in read loop? (kinetic)" class="Bool (strict)"("Value"=w521) -> ()  [unwired: 2 in, 2 out]
                      }
                    }
                  }
                }
              }
              n235 = while {
                shift-right: [w647] -> _
                shift-left: w404 -> [w648]
                shift-right: [w639] -> _
                shift-left: OSPEC-enum."Wait" -> [w649]
                shift-right: [w646] -> w421
                shift-left: w410 -> [w645]
                shift-right: [w640] -> w420
                shift-left: w411 -> [w643]
                shift-right: [w642] -> _
                shift-left: w417 -> [w641]
                shift-right: [w637] -> w413
                shift-left: w406 -> [w638]
                i -> [w644]
                stop <- w634 stop-if-true
                n236 = case shown="\"Read\", Default" w649 {
                  tunnel: w648 -> [w655 w665 w681]
                  tunnel: [w655 w665 w681] -> w647
                  tunnel: [w653 FALSE FALSE] -> w636
                  tunnel: [w659 w669 w679] -> w646
                  tunnel: w645 -> [w659 w670 w679]
                  tunnel: w644 -> [_ w674 _]
                  tunnel: [w657 w673 w676] -> w640
                  tunnel: w643 -> [w657 w672 w676]
                  tunnel: [w654 w666 w678] -> w642
                  tunnel: w641 -> [w654 _ w678]
                  tunnel: [OSPEC-enum."Wait" OSPEC-enum."Check exit" OSPEC-enum."Read"] -> w639
                  tunnel: w638 -> [w656 w662 w675]
                  tunnel: [w656 w661 w675] -> w637
                  frame "Check exit" {
                    n237 = Unbundle By Name(w655) -> ("V off time"=w651:dbl)
                    n238 = Multiply(x=w651, y=1000.0) -> (x*y=w652:dbl)
                    n239 = Greater Or Equal?(x=w654, y=w652) -> (x >= y?=w653:bool)
                  }
                  frame "Read", Default {
                    # "Building a 1d matrix of potentials and times"
                    n240 = call "IV getpotential.vi"("error in (no error)"=w662) -> ("error out"=w661:errorcluster, "value out"=w663:dbl)  [unwired: 8 in, 1 out]
                    "OCP" <- w663
                    n241 = Unbundle By Name(w665) -> ("Start time"=w664:i32)
                    n242 = Tick Count (ms)() -> (millisecond timer value=w660:u32)
                    n243 = Subtract(x=w660, y=w664) -> (x-y=w666:u32)
                    n244 = Equal?(x=1, y=w674) -> ()  [unwired: 1 out]
                    n245 = Build Array (concatenate)(w672, w663) -> (w673:dbl[])
                    n246 = Build Array (concatenate)(w670, w666) -> (w669:u32[])
                  }
                  frame "Wait" {
                    n247 = Unbundle By Name(w681) -> ("Sample rate"=w682:dbl)
                    n248 = Multiply(x=w682, y=1000.0) -> (x*y=w684:dbl)
                    n249 = Wait (ms)(milliseconds to wait=w684) -> ()  [unwired: 1 out]
                  }
                }
                n250 = property on="IDus not in read loop? (kinetic)" class="Bool (strict)"() -> ("Value"=w635:bool)  [unwired: 2 in, 2 out]
                n251 = And(x=w635, y=w636) -> (x .and. y?=w634:bool)
              }
              n252 = Bundle By Name(cluster=w404, "Time for spectrum measurment"=w422, "Time elapsed"=w423, "Spectrum"=w412) -> (w419:T10)
              n253 = Bundle By Name(cluster=w419, "Time for E measurment"=w421, "Potential array"=w420) -> (w414:T10)
            }
            frame "Read current and spectrum" {
              n254 = local read "V (during measurment)"() -> (w697:dbl)
              n255 = Unbundle By Name(w689) -> ("Time for spectrum measurment"=w690:i32[], "Start time"=w696:i32)
              n256 = Unbundle By Name(w689) -> ("V 1"=w698:dbl, "Spectrum"=w693:dbl[][])
              n257 = property on="Use iDus?" class="Bool (strict)"() -> ("Value"=w686:bool)  [unwired: 2 in, 2 out]
              n258 = Equal?(x=w697, y=w698) -> (x = y?=w694:bool)
              n259 = case shown="True" w686 {
                tunnel: [w723 w811] -> w704
                tunnel: [w722 w813] -> w703
                tunnel: [w711 w810] -> w702
                tunnel: w696 -> [w721 w812]
                tunnel: w694 -> [w720 w816]
                tunnel: w693 -> [w715 w817]
                tunnel: w690 -> [w714 w815]
                tunnel: w689 -> [w713 w814]
                frame False {
                  (unwired) FALSE
                  n260 = Unbundle By Name(w713) -> ("Continous strobe delay"=w719:i32, "Integration time"=w718:i32)  [unwired: 1 out]
                  n261 = call "Initalise spectrometer.vi"("Continous strobe delay"=w719, "Enter the \nInetegration Time"=w718) -> ("Wrapper Out"=w712:u32, "ContinuousStrobe Out"=w717:u32, "WL Values"=w716:dbl[])  [unwired: 7 in]
                  "ContinuousStrobe Out" <- w717
                  "Wrapper Out" <- w712
                  "WL Values" <- w716
                  n262 = while {
                    shift-right: [w740] -> _
                    shift-left: w713 -> [w741]
                    shift-right: [w732] -> _
                    shift-left: OSPEC-enum."Wait" -> [w742]
                    shift-right: [w738] -> w711
                    shift-left: w714 -> [w737]
                    shift-right: [w730] -> w722
                    shift-left: w715 -> [w736]
                    shift-right: [w735] -> w723
                    shift-left: w721 -> [w734]
                    tunnel: w720 -> [w731]
                    tunnel: w712 -> [w729]
                    tunnel: [w728] -> _
                    tunnel: w717 -> [w727]
                    tunnel: w716 -> [w726]
                    tunnel: [w725] -> _
                    i -> [w733]
                    stop <- w739 stop-if-true
                    n263 = case shown="\"Read\", Default" w742 {
                      tunnel: w741 -> [w751 w767 w806]
                      tunnel: [w750 w767 w806] -> w740
                      tunnel: [w748 FALSE FALSE] -> w739
                      tunnel: [w752 w786 w804] -> w738
                      tunnel: w737 -> [w752 w785 w804]
                      tunnel: w733 -> [_ w780 _]
                      tunnel: [w743 w773 w799] -> w730
                      tunnel: w736 -> [w743 w784 w799]
                      tunnel: [w749 w775 w803] -> w735
                      tunnel: w734 -> [w749 _ w803]
                      tunnel: [OSPEC-enum."Wait" OSPEC-enum."Check exit" OSPEC-enum."Read"] -> w732
                      tunnel: w731 -> [w746 w779 _]
                      tunnel: w729 -> [w744 w771 w800]
                      tunnel: [w745 w772 w801] -> w728
                      tunnel: w727 -> [w745 w772 w801]
                      tunnel: w726 -> [_ w770 _]
                      tunnel: [w744 w771 w800] -> w725
                      frame "Check exit" {
                        n264 = case shown="True" w746 {
                          tunnel: w751 -> [w758 w764]
                          tunnel: [w758 w764] -> w750
                          tunnel: w749 -> [w756 w762]
                          tunnel: [w757 w763] -> w748
                          frame False {
                            n265 = Unbundle By Name(w758) -> ("V2 time"=w755:dbl)
                            n266 = Multiply(x=w755, y=1000.0) -> (x*y=w753:dbl)
                            n267 = Greater Or Equal?(x=w756, y=w753) -> (x >= y?=w757:bool)
                          }
                          frame True {
                            n268 = Unbundle By Name(w764) -> ("V1 time"=w761:dbl)
                            n269 = Multiply(x=w761, y=1000.0) -> (x*y=w759:dbl)
                            n270 = Greater Or Equal?(x=w762, y=w759) -> (x >= y?=w763:bool)
                          }
                        }
                      }
                      frame "Read", Default {
                        # "Check here to see if DIM t + 1 and DIM WL match"
                        n271 = Tick Count (ms)() -> (millisecond timer value=w765:u32)
                        n272 = call "Wrapper_getSpectrum.vi"("Index"=0, "Wrapper"=w771) -> ("Spectrum Values"=w769:dbl[])  [unwired: 1 out]
                        n273 = Unbundle By Name(w767) -> ("Start time"=w766:i32)
                        n274 = Subtract(x=w765, y=w766) -> (x-y=w776:u32)
                        n275 = Bundle("WL Values"=w770, "Spectrum Values"=w769) -> (→"?":T4)  [unwired: 1 in]
                        n276 = Equal?(x=w780, y=1.0) -> (x = y?=w778:bool)
                        n277 = And(x=w779, y=w778) -> (x .and. y?=w777:bool)
                        n278 = case shown="True" w777 {
                          tunnel: [w789 w790] -> w773
                          tunnel: w784 -> [w788 _]
                          tunnel: w769 -> [w787 w792]
                          tunnel: w770 -> [_ w791]
                          frame False {
                            # "Intensity thereafter"
                            n279 = Build Array (concatenate)(w788, w787) -> (w789:dbl[][])
                          }
                          frame True {
                            n280 = Build Array(w791, w792) -> (w790:dbl[][])
                          }
                        }
                        n281 = case shown="True" w777 {
                          tunnel: [w795 w798] -> w786
                          tunnel: w785 -> [w794 w797]
                          tunnel: w776 -> [w793 w796]
                          tunnel: [w793 w796] -> w775
                          frame False {
                            n282 = Build Array (concatenate)(w794, w793) -> (w795:u32[])
                          }
                          frame True {
                            n283 = Build Array (concatenate)(w797, w796) -> (w798:u32[])
                          }
                        }
                      }
                      frame "Wait" {
                        n284 = Unbundle By Name(w806) -> ("Sample rate"=w807:dbl)
                        n285 = Multiply(x=w807, y=1000.0) -> (x*y=w809:dbl)
                        n286 = Wait (ms)(milliseconds to wait=w809) -> ()  [unwired: 1 out]
                      }
                    }
                  }
                }
                frame True {
                  n287 = while {
                    shift-right: [w829] -> w811
                    shift-left: w812 -> [w830]
                    shift-right: [w822] -> _
                    shift-left: OSPEC-enum."Wait" -> [w831]
                    shift-right: [w828] -> w810
                    shift-left: w815 -> [w827]
                    shift-right: [w820] -> w813
                    shift-left: w817 -> [w826]
                    shift-right: [w825] -> _
                    shift-left: w814 -> [w824]
                    tunnel: w816 -> [w821]
                    i -> [w823]
                    stop <- w819 stop-if-true
                    n288 = case shown="\"Read\", Default" w831 {
                      tunnel: w830 -> [w839 _ w967]
                      tunnel: [w838 w855 w967] -> w829
                      tunnel: [w836 FALSE FALSE] -> w819
                      tunnel: [w840 w856 w965] -> w828
                      tunnel: w827 -> [w840 w861 w965]
                      tunnel: w823 -> [_ w865 _]
                      tunnel: w826 -> [w833 w859 w961]
                      tunnel: [w837 w854 w963] -> w825
                      tunnel: w824 -> [w837 w854 w963]
                      tunnel: [OSPEC-enum."Wait" OSPEC-enum."Check exit" OSPEC-enum."Read"] -> w822
                      tunnel: w821 -> [w834 w860 _]
                      tunnel: [w833 w857 w961] -> w820
                      frame "Check exit" {
                        n289 = case shown="False" w834 {
                          tunnel: w839 -> [w842 w847]
                          tunnel: [w842 w847] -> w838
                          tunnel: w837 -> [w841 w848]
                          tunnel: [w846 w852] -> w836
                          frame False {
                            n290 = Unbundle By Name(w841) -> ("V2 time"=w843:dbl)
                            n291 = Multiply(x=w843, y=1000.0) -> (x*y=w844:dbl)
                            n292 = Greater Or Equal?(x=w842, y=w844) -> (x >= y?=w846:bool)
                          }
                          frame True {
                            n293 = Unbundle By Name(w848) -> ("V1 time"=w849:dbl)
                            n294 = Multiply(x=w849, y=1000.0) -> (x*y=w850:dbl)
                            n295 = Greater Or Equal?(x=w847, y=w850) -> (x >= y?=w852:bool)
                          }
                        }
                      }
                      frame "Read", Default {
                        n296 = Unbundle By Name(w854) -> ("Start time"=w853:i32)
                        n297 = property on="Number of scans in kinetic cycle" class="DigNum (strict)"() -> ("Value"=w864:i32)  [unwired: 2 in, 2 out]
                        n298 = Tick Count (ms)() -> (millisecond timer value=w862:u32)
                        n299 = Subtract(x=w862, y=w853) -> (x-y=w855:u32)
                        n300 = call "GetDetector.vi"() -> ("xpixels"=w863:i32)  [unwired: 4 in, 3 out]
                        n301 = Equal?(x=w865, y=1.0) -> (x = y?=w858:bool)
                        n302 = stacked-sequence {
                          seq-local: [_ _ _ _ _ _ _ _ _ _ w899 _] -> [_ _ _ _ _ _ _ _ _ _ _ w920]
                          seq-local: [_ _ _ _ _ _ _ _ w884 _ _ _] -> [_ _ _ _ _ _ _ _ _ _ _ w918]
                          seq-local: [_ _ _ _ _ _ _ _ _ _ w898 _] -> [_ _ _ _ _ _ _ _ _ _ _ w919]
                          tunnel: [_ _ _ _ _ _ _ _ _ _ _ w913] -> w857
                          tunnel: [_ _ _ _ _ _ _ _ _ _ _ w914] -> w856
                          tunnel: w864 -> [_ _ _ _ _ w877 _ _ _ _ w895 w912]
                          tunnel: w855 -> [_ _ _ _ _ _ _ _ _ _ _ w915]
                          tunnel: w863 -> [_ w870 _ _ _ _ _ _ _ _ _ _]
                          tunnel: w853 -> [_ _ _ _ _ _ _ _ w883 _ w897 _]
                          tunnel: w861 -> [_ _ _ _ _ _ _ _ _ _ _ w911]
                          tunnel: w860 -> [_ _ _ _ _ _ _ _ _ _ _ w910]
                          tunnel: w859 -> [_ _ _ _ _ _ _ _ _ _ _ w909]
                          tunnel: w858 -> [_ _ _ _ _ _ _ _ _ _ _ w908]
                          frame #0 {
                            w869 = u16 3  # AcquisitionMode
                            n303 = call "SetAcquisitionMode.vi"("mode"=w869) -> ()  [unwired: 1 in, 2 out]
                          }
                          frame #1 {
                            w871 = u16 0  # ReadMode
                            n304 = property on="xpixels" class="DigNum (strict)"("Value"=w870) -> ()  [unwired: 2 in, 2 out]
                            n305 = call "SetReadMode.vi"("mode"=w871) -> ()  [unwired: 1 in, 2 out]
                          }
                          frame #2 {
                            n306 = call "SetTriggerMode.vi"("mode"=TriggerMode_mode_typedef."Internal") -> ()  [unwired: 1 in, 2 out]
                          }
                          frame #3 {
                            n307 = property on="Exposure time (s)" class="DigNum (strict)"() -> ("Value"=w873:dbl)  [unwired: 2 in, 2 out]
                            n308 = call "SetExposureTime.vi"("time"=w873) -> ()  [unwired: 1 in, 2 out]
                          }
                          frame #4 {
                            n309 = call "GetNumberVSSpeeds.vi"() -> ("number"=w876:i32)  [unwired: 3 in, 2 out]
                            n310 = Subtract(x=w876, y=1) -> (x-y=w874:i32)
                            n311 = call "SetVSSpeed.vi"("index"=w874) -> ()  [unwired: 1 in, 2 out]
                          }
                          frame #5 {
                            n312 = call "SetNumberKinetics.vi"("number"=w877) -> ()  [unwired: 1 in, 2 out]
                          }
                          frame #6 {
                            w880 = 0  # Auto Shutter
                            n313 = call "SetShutter.vi"("type"="Shutter opens on TTL", "mode"=w880, "closingtime"="Shutter open and close time", "openingtime"="Shutter open and close time") -> ()  [unwired: 10 in, 2 out]
                          }
                          frame #7 {
                            # "Meybe delete the exposure time insupt here"
                            n314 = property on="Exposure time (s)" class="DigNum (strict)"() -> ("Value"=w881:dbl)  [unwired: 2 in, 2 out]
                            n315 = call "GetAcquisitionTimings.vi"("exposure input"=w881) -> ("exposure"=w882:sgl)  [unwired: 10 in, 4 out]
                            n316 = property on="Calculated exposure time" class="DigNum (strict)"("Value"=w882) -> ()  [unwired: 2 in, 2 out]
                          }
                          frame #8 {
                            n317 = flat-sequence {
                              tunnel: [w886] -> w884
                              tunnel: w883 -> [w885]
                              frame #0 {
                                n318 = Tick Count (ms)() -> (millisecond timer value=w887:u32)
                                n319 = Subtract(x=w887, y=w885) -> (x-y=w886:u32)
                                "Time before the start of current aquisition (ms)" <- w886
                              }
                              frame #1 {
                                n320 = call "StartAcquisition.vi"() -> ("DLL error code"=w888:u32)  [unwired: 2 in, 1 out]
                                n321 = property on="Start Aquisition return code" class="DigNum (strict)"("Value"=w888) -> ()  [unwired: 2 in, 2 out]
                              }
                            }
                          }
                          frame #9 {
                            n322 = while {
                              stop <- w892 continue-if-true
                              w893 = u16 72  # DRV ACQUIRING
                              n323 = call "GetStatus.vi"() -> ("DLL error code"=w890:u32, "status"=w891:T17)  [unwired: 3 in, 1 out]
                              n324 = property on="Get status return code" class="DigNum (strict)"("Value"=w890) -> ()  [unwired: 2 in, 2 out]
                              n325 = Equal?(x=w891, y=w893) -> (x = y?=w892:bool)
                              "IDus not in read loop? (kinetic)" <- FALSE
                            }
                          }
                          frame #10 {
                            n326 = flat-sequence {
                              tunnel: [w900] -> w898
                              tunnel: w897 -> [w901]
                              tunnel: [w907] -> w899
                              tunnel: w896 -> [w903]
                              frame #0 {
                                n327 = Tick Count (ms)() -> (millisecond timer value=w902:u32)
                                n328 = Subtract(x=w902, y=w901) -> (x-y=w900:u32)
                                "Time  after the aquisition (before fetch data), (ms)" <- w900
                              }
                              frame #1 {
                                n329 = call "GetAcquiredData.vi"("size"=w903) -> ("DLL error code"=w904:u32, "array"=w907:i32[])  [unwired: 2 in, 1 out]
                                n330 = Equal?(x=20002 ("DRV_SUCCESS"), y=w904) -> (x = y?=→"Get aqisition ok? (kinetic mode)":bool)
                                n331 = property on="get aquired data return code" class="DigNum (strict)"("Value"=w904) -> ()  [unwired: 2 in, 2 out]
                              }
                            }
                            n332 = Multiply(x=1024, y=w895) -> (x*y=w896:i32)
                          }
                          frame #11 {
                            n333 = Subtract(x=w919, y=w918) -> (x-y=w917:u32)
                            n334 = Divide(x=w917, y=w912) -> (x/y=w916:dbl)
                            n335 = for {
                              N: w912 -> [_]
                              tunnel: w920 -> [w938]
                              tunnel: w916 -> [w936]
                              tunnel: w915 -> [w933]
                              shift-right: [w931] -> w913
                              shift-left: w909 -> [w930]
                              shift-right: [w923] -> w914
                              shift-left: w911 -> [w928]
                              tunnel: w910 -> [w926]
                              tunnel: w908 -> [w924]
                              i -> [w922]
                              w932 = 1024 ("x")
                              n336 = Equal To 0?(x=w922) -> (x = 0?=w921:bool)
                              n337 = Multiply(x=w922, y=w936) -> (x*y=w935:dbl)
                              n338 = Multiply(x=w932, y=w922) -> (x*y=w937:i32)
                              n339 = Add(x=w935, y=w933) -> (x+y=w929:dbl)
                              n340 = Array Subset(array=w938, index=w937, length=w932) -> (w934:i32[])
                              n341 = And(x=w921, y=w924) -> (x .and. y?=w925:bool)
                              n342 = And(x=w926, y=w925) -> (x .and. y?=w927:bool)
                              n343 = case shown="False" w927 {
                                tunnel: w934 -> [w939 w952]
                                tunnel: [w944 w955] -> w931
                                tunnel: w930 -> [w945 _]
                                tunnel: w929 -> [w942 w957]
                                tunnel: [w941 w956] -> w923
                                tunnel: w928 -> [w943 _]
                                tunnel: w921 -> [w940 _]
                                frame False {
                                n344 = case shown="True" w940 {
                                tunnel: w939 -> [_ w948]
                                frame False {
                                }
                                frame True {
                                n345 = for {
                                N: 1023 -> [_]
                                tunnel: [w950] -> _ mode=indexing
                                tunnel: [w950] -> w947 mode=indexing
                                i -> [w951]
                                n346 = Increment(x=w951) -> (x+1=w950:i32)
                                }
                                n347 = Bundle(w947, w948) -> (w946:cluster{i32[], i32[]})  [unwired: 1 in]
                                n348 = property class="XYGraph (strict)"("Value"=w946) -> ()  [unwired: 2 in, 2 out]
                                }
                                }
                                n349 = Build Array (concatenate)(w945, w939) -> (w944:dbl[][])
                                n350 = Build Array (concatenate)(w943, w942) -> (w941:dbl[])
                                }
                                frame True {
                                n351 = for {
                                N: 1023 -> [_]
                                tunnel: [w959] -> w953 mode=indexing
                                i -> [w960]
                                n352 = Increment(x=w960) -> (x+1=w959:i32)
                                }
                                n353 = Bundle(w953, w952) -> (w954:cluster{i32[], i32[]})  [unwired: 1 in]
                                n354 = Build Array(w957) -> (w956:dbl[])
                                n355 = Build Array(w953, w952) -> (w955:i32[][])
                                n356 = property class="XYGraph (strict)"("Value"=w954) -> ()  [unwired: 2 in, 2 out]
                                }
                              }
                            }
                          }
                        }
                      }
                      frame "Wait" {
                        n357 = Unbundle By Name(w963) -> ("Sample rate"=w962:dbl)
                        n358 = Multiply(x=w962, y=1000.0) -> (x*y=w969:dbl)
                        n359 = Wait (ms)(milliseconds to wait=w969) -> ()  [unwired: 1 out]
                      }
                    }
                    n360 = case shown="True" w819 {
                      frame False {
                      }
                      frame True {
                        n361 = property on="IDus not in read loop? (kinetic)" class="Bool (strict)"("Value"=TRUE ("IDus not in read loop? (kinetic)")) -> ()  [unwired: 2 in, 2 out]
                      }
                    }
                  }
                }
              }
              n362 = Unbundle By Name(w689) -> ("Current array"=w688:dbl[])
              n363 = Unbundle By Name(w689) -> ("Time for I measurment"=w687:i32[], "Start time"=w695:i32)
              n364 = while {
                shift-right: [w984] -> _
                shift-left: w689 -> [w985]
                shift-right: [w976] -> _
                shift-left: OSPEC-enum."Wait" -> [w986]
                shift-right: [w983] -> w701
                shift-left: w687 -> [w982]
                shift-right: [w977] -> w685
                shift-left: w688 -> [w980]
                shift-right: [w979] -> _
                shift-left: w695 -> [w978]
                tunnel: w694 -> [w975]
                shift-right: [w973] -> w691
                shift-left: w692 -> [w974]
                i -> [w981]
                stop <- w970 stop-if-true
                n365 = case shown="\"Check exit\"" w986 {
                  tunnel: w985 -> [w995 w1014 w1051]
                  tunnel: [w994 w1014 w1051] -> w984
                  tunnel: [w992 FALSE FALSE] -> w971
                  tunnel: [w997 w1025 w1049] -> w983
                  tunnel: w982 -> [w997 w1026 w1049]
                  tunnel: w981 -> [_ w1031 _]
                  tunnel: [w989 w1030 w1046] -> w977
                  tunnel: w980 -> [w989 w1029 w1046]
                  tunnel: [w987 w1015 w1048] -> w979
                  tunnel: w978 -> [w987 _ w1048]
                  tunnel: [OSPEC-enum."Wait" OSPEC-enum."Check exit" OSPEC-enum."Read"] -> w976
                  tunnel: w975 -> [_ w1020 _]
                  tunnel: w974 -> [w988 w1012 w1045]
                  tunnel: [w988 w1011 w1045] -> w973
                  frame "Check exit" {
                    n366 = local read "V (during measurment)"() -> (w991:dbl)
                    n367 = Unbundle By Name(w995) -> ("V 1"=w996:dbl)
                    n368 = Equal?(x=w996, y=w991) -> (x = y?=w993:bool)
                    n369 = case shown="True" w993 {
                      tunnel: w995 -> [w1003 w1009]
                      tunnel: [w1003 w1009] -> w994
                      tunnel: [w1002 w1008] -> w992
                      tunnel: w987 -> [w1001 w1007]
                      frame False {
                        n370 = Unbundle By Name(w1003) -> ("V2 time"=w999:dbl)
                        n371 = Multiply(x=1000.0, y=w999) -> (x*y=w1000:dbl)
                        n372 = Greater Or Equal?(x=w1001, y=w1000) -> (x >= y?=w1002:bool)
                      }
                      frame True {
                        n373 = Unbundle By Name(w1009) -> ("V1 time"=w1005:dbl)
                        n374 = Multiply(x=w1005, y=1000.0) -> (x*y=w1006:dbl)
                        n375 = Greater Or Equal?(x=w1007, y=w1006) -> (x >= y?=w1008:bool)
                      }
                    }
                  }
                  frame "Read", Default {
                    # "Building a 1d matrix of currents"
                    n376 = call "IV getcurrent.vi"("error in (no error)"=w1012) -> ("error out"=w1017:errorcluster, "value out"=w1018:dbl)  [unwired: 8 in, 1 out]
                    n377 = flat-sequence {
                      tunnel: w1018 -> [w1033]
                      tunnel: w1017 -> [w1032]
                      tunnel: [w1032] -> w1016
                      frame #0 {
                        n378 = call "Current ranging routine (SubVI).vi"("Current"=w1033) -> ()  [unwired: 11 in]
                      }
                    }
                    n379 = Unbundle By Name(w1014) -> ("Start time"=w1013:i32)
                    n380 = call "IV getcurrent.vi"("error in (no error)"=w1016) -> ("error out"=w1011:errorcluster, "value out"=w1024:dbl)  [unwired: 8 in, 1 out]
                    n381 = Tick Count (ms)() -> (millisecond timer value=w1010:u32)
                    n382 = Subtract(x=w1010, y=w1013) -> (x-y=w1027:u32)
                    n383 = Equal?(x=1, y=w1031) -> (x = y?=w1021:bool)
                    n384 = And(x=w1020, y=w1021) -> (x .and. y?=w1019:bool)
                    n385 = case shown="True" w1019 {
                      tunnel: [w1035 w1039] -> w1025
                      tunnel: w1026 -> [w1036 w1037]
                      tunnel: w1027 -> [w1034 w1038]
                      tunnel: [w1034 w1038] -> w1015
                      frame False {
                        n386 = Build Array (concatenate)(w1036, w1034) -> (w1035:u32[])
                      }
                      frame True {
                        n387 = Build Array (concatenate)(w1037, w1038) -> (w1039:u32[])
                      }
                    }
                    n388 = case shown="False" w1019 {
                      tunnel: [w1041 w1043] -> w1030
                      tunnel: w1029 -> [w1042 _]
                      tunnel: w1024 -> [w1040 w1044]
                      frame False {
                        # "Intensity thereafter"
                        n389 = Build Array (concatenate)(w1042, w1040) -> (w1041:dbl[])
                      }
                      frame True {
                        n390 = Build Array(w1044) -> (w1043:dbl[])
                      }
                    }
                  }
                  frame "Wait" {
                    n391 = Unbundle By Name(w1051) -> ("Sample rate"=w1052:dbl)
                    n392 = Multiply(x=w1052, y=1000.0) -> (x*y=w1054:dbl)
                    n393 = Wait (ms)(milliseconds to wait=w1054) -> ()  [unwired: 1 out]
                  }
                }
                n394 = property on="IDus not in read loop? (kinetic)" class="Bool (strict)"() -> ("Value"=w972:bool)  [unwired: 2 in, 2 out]
                n395 = And(x=w972, y=w971) -> (x .and. y?=w970:bool)
              }
              n396 = Bundle By Name(cluster=w689, "Time for spectrum measurment"=w702, "Time elapsed"=w704, "Spectrum"=w703) -> (w699:T10)
              n397 = Bundle By Name(cluster=w699, "Time for I measurment"=w701, "Current array"=w685) -> (w700:T10)
              n398 = local read "V (during measurment)"() -> (w706:dbl)
              n399 = Unbundle By Name(w699) -> ("V 1"=w707:dbl)
              n400 = Equal?(x=w707, y=w706) -> (x = y?=w708:bool)
              n401 = case shown="True" w708 {
                tunnel: [OSSPEC."Read Potential and spectrum" OSSPEC."Apply V2"] -> w709
                frame False {
                }
                frame True {
                }
              }
            }
            frame "Reinitialise Cell" {
              # "this state is no longer used as it adds a 1-300 ms delay before the spectrum is measured as the mode is shifted"
              n402 = flat-sequence {
                tunnel: w1063 -> [w1067]
                tunnel: [w1066] -> w1058
                tunnel: w1058 -> [w1070]
                tunnel: [w1069] -> w1057
                tunnel: [w1071] -> w1062
                tunnel: w1057 -> [w1071]
                frame #0 {
                  n403 = To Long Integer(number=T16."IStat4EL" ("Configuration")) -> (32bit integer=w1065:i32)
                  n404 = call "IV setconnectionmode.vi"("error in (no error)"=w1067, "value"=w1065) -> ("error out"=w1066:errorcluster)  [unwired: 7 in, 2 out]
                }
                frame #1 {
                  n405 = call "IV setcurrent.vi"("error in (no error)"=w1070, "value"=0.0) -> ("error out"=w1069:errorcluster)  [unwired: 7 in, 2 out]
                }
                frame #2 {
                }
              }
              n406 = Unbundle By Name(w1059) -> ()  [unwired: 3 out]
            }
            frame "Apply V1" {
              n407 = flat-sequence {
                tunnel: w1082 -> [w1087]
                tunnel: [w1088] -> w1083
                tunnel: w1077 -> [w1086]
                tunnel: [w1085] -> w1073
                tunnel: w1083 -> [w1103]
                tunnel: w1082 -> [w1101]
                tunnel: [w1102] -> w1081
                tunnel: [w1100] -> w1079
                tunnel: w1073 -> [w1098]
                tunnel: w1081 -> [w1106]
                tunnel: [w1106] -> w1080
                tunnel: w1079 -> [w1105]
                tunnel: [w1105] -> w1078
                tunnel: w1080 -> [w1109]
                tunnel: w1078 -> [w1107]
                tunnel: [w1108] -> w1072
                tunnel: [w1107] -> w1074
                frame #0 {
                  n408 = Unbundle By Name(w1087) -> ("V 1"=w1085:dbl)
                  n409 = Absolute Value(x=w1085) -> (abs(x)=w1090:dbl)
                  n410 = local write "V (during measurment)"(w1085) -> ()
                  n411 = Greater?(x=w1090, y=3.0) -> (0:w1089:bool)
                  n412 = case shown="True" w1089 {
                    tunnel: [w1091 w1093] -> w1088
                    tunnel: w1086 -> [w1091 w1092]
                    frame False {
                    }
                    frame True {
                      # "abort if E >3 V"
                      n413 = call "IV setcellon.vi"("error in (no error)"=w1092, "cellon"=0) -> ("error out"=w1095:errorcluster)  [unwired: 7 in, 2 out]
                      n414 = call "IV close.vi"("error in (no error)"=w1095) -> ("error out"=w1093:errorcluster)  [unwired: 9 in, 1 out]
                      n415 = call "Display Message to User3"("error in (no error)"=w1093) -> ("OK"=w1096:bool)  [unwired: 9 in, 1 out]
                      n416 = Stop(stop? (T)=w1096) -> ()
                    }
                  }
                }
                frame #1 {
                  n417 = call "IV setpotential.vi"("error in (no error)"=w1103, "value"=w1098) -> ("error out"=w1102:errorcluster)  [unwired: 7 in, 2 out]
                  n418 = Tick Count (ms)() -> (millisecond timer value=w1097:u32)
                  n419 = Bundle By Name(cluster=w1101, "Start time"=w1097, "Time elapsed"=0) -> (w1100:T10)
                }
                frame #2 {
                  n420 = Wait (ms)(milliseconds to wait=u32 100) -> ()  [unwired: 1 out]
                }
                frame #3 {
                  n421 = call "IV getcurrent.vi"("error in (no error)"=w1109) -> ("error out"=w1108:errorcluster, "value out"=w1110:dbl)  [unwired: 8 in, 1 out]
                  n422 = call "Current ranging routine (SubVI).vi"("Current"=w1110) -> ()  [unwired: 11 in]
                }
              }
            }
            frame "Apply V2" {
              n423 = Tick Count (ms)() -> (millisecond timer value=w1114:u32)
              n424 = flat-sequence {
                tunnel: w1119 -> [w1130]
                tunnel: [w1131] -> w1126
                tunnel: w1122 -> [w1129]
                tunnel: [w1128] -> w1118
                tunnel: [w1127] -> w1115
                tunnel: w1114 -> [w1127]
                tunnel: w1126 -> [w1144]
                tunnel: [w1143] -> w1125
                tunnel: w1118 -> [w1142]
                tunnel: [w1141] -> w1116
                tunnel: w1115 -> [w1141]
                tunnel: w1125 -> [w1147]
                tunnel: [w1147] -> w1124
                tunnel: [w1145] -> w1117
                tunnel: w1116 -> [w1145]
                tunnel: w1124 -> [w1150]
                tunnel: [w1149] -> w1123
                tunnel: [w1148] -> w1112
                tunnel: w1117 -> [w1148]
                frame #0 {
                  n425 = Unbundle By Name(w1130) -> ("V 2"=w1128:dbl)
                  n426 = Absolute Value(x=w1128) -> (abs(x)=w1134:dbl)
                  n427 = local write "V (during measurment)"(w1128) -> ()
                  n428 = Greater?(x=w1134, y=3.0) -> (0:w1132:bool)
                  n429 = case shown="False" w1132 {
                    tunnel: [w1135 w1137] -> w1131
                    tunnel: w1129 -> [w1135 w1136]
                    frame False {
                    }
                    frame True {
                      # "abort if E >3 V"
                      n430 = call "IV setcellon.vi"("error in (no error)"=w1136, "cellon"=0) -> ("error out"=w1139:errorcluster)  [unwired: 7 in, 2 out]
                      n431 = call "IV close.vi"("error in (no error)"=w1139) -> ("error out"=w1137:errorcluster)  [unwired: 9 in, 1 out]
                      n432 = call "Display Message to User4"("error in (no error)"=w1137) -> ("OK"=w1140:bool)  [unwired: 9 in, 1 out]
                      n433 = Stop(stop? (T)=w1140) -> ()
                    }
                  }
                }
                frame #1 {
                  n434 = call "IV setpotential.vi"("error in (no error)"=w1144, "value"=w1142) -> ("error out"=w1143:errorcluster)  [unwired: 7 in, 2 out]
                }
                frame #2 {
                  n435 = Wait (ms)(milliseconds to wait=u32 100) -> ()  [unwired: 1 out]
                }
                frame #3 {
                  n436 = call "IV getcurrent.vi"("error in (no error)"=w1150) -> ("error out"=w1149:errorcluster, "value out"=w1151:dbl)  [unwired: 8 in, 1 out]
                  n437 = call "Current ranging routine (SubVI).vi"("Current"=w1151) -> ()  [unwired: 11 in]
                }
              }
              n438 = Tick Count (ms)() -> (millisecond timer value=w1113:u32)
              n439 = Subtract(x=w1112, y=w1113) -> (x-y=→"Time taken to apply V2":u32)
              n440 = Unbundle By Name(w1119) -> ()  [unwired: 3 out]
            }
            frame "End measurment" {
              w1159 = ext 0.00099999999999999999996
              n441 = Unbundle By Name(w1153) -> ("Time for spectrum measurment"=w1155:i32[], "Spectrum"=w1172:dbl[][])
              n442 = Unbundle By Name(w1153) -> ("Current array"=w1166:dbl[], "Time for I measurment"=w1161:i32[])
              n443 = Unbundle By Name(w1153) -> ("Time for E measurment"=w1158:i32[], "Potential array"=w1167:dbl[])
              n444 = Multiply(x=w1155, y=ext 0.00099999999999999999996) -> (x*y=w1154:ext[])
              n445 = Insert Into Array(array=w1154, index=0, new element=0 ("new element/subarray")) -> (w1170:ext[])
              n446 = Multiply(x=w1159, y=w1158) -> (x*y=w1157:ext[])
              n447 = Multiply(x=w1161, y=w1159) -> (x*y=w1160:ext[])
              n448 = Build Array(w1160, w1166) -> (w1165:ext[][])
              n449 = Build Array(w1157, w1167) -> (w1163:ext[][])
              n450 = Insert Into Array(array=w1172, index (col)=0 ("disabled index (col)"), new element=w1170) -> (w1169:dbl[][])  [unwired: 1 in]
              n451 = Transpose 2D Array(2D array=w1163) -> (transposed array=w1162:ext[][])
              n452 = Transpose 2D Array(2D array=w1165) -> (transposed array=w1164:ext[][])
              n453 = call "Write-OSP-E-t.vi"("Init cluster"=w1153, "Array"=w1162) -> ()  [unwired: 10 in]
              n454 = Transpose 2D Array(2D array=w1169) -> (transposed array=w1168:dbl[][])
              n455 = call "Write-OSP-J-t.vi"("Init cluster"=w1153, "Array"=w1164) -> ()  [unwired: 10 in]
              n456 = call "Write-OSP-SP.vi"("Init cluster"=w1153, "Array"=w1168) -> ()  [unwired: 10 in]
              n457 = property on="T reached?" class="Bool (strict)"("Value"=FALSE ("T reached?")) -> ()  [unwired: 2 in, 2 out]
              n458 = flat-sequence {
                tunnel: w1180 -> [w1183]
                tunnel: [w1182] -> w1179
                tunnel: w1181 -> [w1188]
                tunnel: w1179 -> [w1187]
                tunnel: [w1186] -> w1176
                tunnel: w1176 -> [w1190]
                tunnel: [w1189] -> w1175
                frame #0 {
                  n459 = To Long Integer(number=T16."EStat4EL" ("Configuration")) -> (32bit integer=w1185:i32)
                  n460 = call "IV setconnectionmode.vi"("error in (no error)"=w1183, "value"=w1185) -> ("error out"=w1182:errorcluster)  [unwired: 7 in, 2 out]
                }
                frame #1 {
                  n461 = call "IV setpotential.vi"("error in (no error)"=w1187, "value"=w1188) -> ("error out"=w1186:errorcluster)  [unwired: 7 in, 2 out]
                }
                frame #2 {
                  n462 = call "IV getcurrent.vi"("error in (no error)"=w1190) -> ("error out"=w1189:errorcluster, "value out"=w1191:dbl)  [unwired: 8 in, 1 out]
                  n463 = call "Current ranging routine (SubVI).vi"("Current"=w1191) -> ()  [unwired: 11 in]
                }
              }
              n464 = Unbundle By Name(w1153) -> ("Default\n potential"=w1181:dbl)
            }
          }
        }
      }
      frame "Initialse and cool iDus" {
        # "Also re-intialise constants"
        n465 = Unbundle By Name(w1197) -> ("Return detector to \nroom T"=w1200:bool)
        n466 = case shown="False" w1200 {
          tunnel: [State."Wait for Event" ("f") State."Wait for Event" ("f")] -> w1199
          frame False {
            w1209 = 20002  # DRV_SUCCESS
            n467 = stacked-sequence {
              seq-local: [_ _ _ _ _ _ w1275] -> [_ _ _ _ _ _ _]
              seq-local: [_ _ _ _ _ _ w1276] -> [_ _ _ _ _ _ _]
              tunnel: w1209 -> [w1265 _ _ _ _ _ _]
              tunnel: [w1264 _ _ _ _ _ _] -> w1208
              tunnel: [_ _ _ _ _ _ w1275] -> _
              tunnel: [_ _ _ _ _ _ w1276] -> w1203
              frame #0 {
                n468 = call "Initialize.vi"("directory (\"\")"="" ("directory (\"\")")) -> ("DLL error code"=w1267:u32)  [unwired: 1 in, 1 out]
                "Init. return code" <- w1267
                n469 = Equal?(x=w1265, y=w1267) -> (x = y?=w1264:bool)
              }
              frame #1 {
                n470 = Wait (ms)(milliseconds to wait=u32 2000) -> ()  [unwired: 1 out]
              }
              frame #2 {
                w1269 = u16 0  # ReadMode
                n471 = call "SetReadMode.vi"("mode"=w1269) -> ()  [unwired: 1 in, 2 out]
              }
              frame #3 {
                w1270 = u16 1  # AcquisitionMode
                n472 = call "SetAcquisitionMode.vi"("mode"=w1270) -> ()  [unwired: 1 in, 2 out]
              }
              frame #4 {
                w1271 = 0
                n473 = call "SetHSSpeed.vi"("index"=w1271, "type"=w1271) -> ()  [unwired: 2 in, 2 out]
              }
              frame #5 {
                n474 = call "GetNumberVSSpeeds.vi"() -> ("number"=w1274:i32)  [unwired: 3 in, 2 out]
                n475 = Subtract(x=w1274, y=1) -> (x-y=w1272:i32)
                n476 = call "SetVSSpeed.vi"("index"=w1272) -> ()  [unwired: 1 in, 2 out]
              }
              frame #6 {
                n477 = call "GetDetector.vi"() -> ("ypixels"=w1275:i32, "xpixels"=w1276:i32)  [unwired: 4 in, 2 out]
                "xpixels" <- w1276
                "ypixels" <- w1275
              }
            }
            n478 = flat-sequence {
              tunnel: w1208 -> [w1260]
              tunnel: [w1259] -> w1207
              frame #0 {
                n479 = case shown="True" w1260 {
                  selector: w1260 -> [w1262 w1263]
                  tunnel: [w1261 w1263] -> w1259
                  frame False {
                    n480 = Not(x=w1262) -> (.not. x?=w1261:bool)
                    n481 = call "Display Message to User5"() -> ()  [unwired: 10 in, 2 out]
                    n482 = Stop(stop? (T)=w1261) -> ()
                  }
                  frame True {
                  }
                }
              }
            }
            n483 = flat-sequence {
              tunnel: w1207 -> [w1216]
              tunnel: [w1214] -> w1204
              tunnel: w1203 -> [w1214]
              tunnel: [w1213] -> _
              frame #0 {
                w1217 = 36  # DRV_TEMP_STABILIZED
                w1218 = 20002  # DRV_SUCCESS
                # "set T ok?"
                # "timings ok?"
                n484 = stacked-sequence {
                  seq-local: [_ _ w1221 _ _ _] -> [_ _ _ _ _ _]
                  seq-local: [_ _ _ w1229 _ _] -> [_ _ _ _ w1233 w1234]
                  tunnel: w1218 -> [_ _ w1223 w1232 _ _]
                  tunnel: "Temperature\n(degrees C)" -> [_ _ _ w1230 _ _]
                  tunnel: w1217 -> [_ _ _ _ _ w1235]
                  tunnel: w1216 -> [_ _ w1222 _ _ _]
                  tunnel: [_ _ _ _ _ w1234] -> w1213
                  frame #0 {
                    n485 = call "SetTriggerMode.vi"("mode"=TriggerMode_mode_typedef."Internal") -> ()  [unwired: 1 in, 2 out]
                  }
                  frame #1 {
                    n486 = property on="Exposure time (s)" class="DigNum (strict)"() -> ("Value"=w1220:dbl)  [unwired: 2 in, 2 out]
                    n487 = call "SetExposureTime.vi"("time"=w1220) -> ()  [unwired: 1 in, 2 out]
                  }
                  frame #2 {
                    n488 = case shown="True" w1222 {
                      tunnel: w1223 -> [_ w1227]
                      tunnel: [FALSE w1228] -> w1221
                      frame False {
                      }
                      frame True {
                        n489 = call "GetAcquisitionTimings.vi"() -> ("exposure"=→"Calculated exposure time":sgl, "DLL error code"=w1226:u32)  [unwired: 11 in, 3 out]
                        "Check timings return code" <- w1226
                        n490 = Equal?(x=w1227, y=w1226) -> (x = y?=w1228:bool)
                      }
                    }
                  }
                  frame #3 {
                    n491 = call "SetTemperature.vi"("temperature"=w1230) -> ("DLL error code"=w1231:u32)  [unwired: 1 in, 1 out]
                    "Set temprature\nreturn code" <- w1231
                    n492 = Equal?(x=w1232, y=w1231) -> (x = y?=w1229:bool)
                  }
                  frame #4 {
                    n493 = case shown="True" w1233 {
                      frame False {
                      }
                      frame True {
                        n494 = call "CoolerON.vi"() -> ()  [unwired: 2 in, 2 out]
                      }
                    }
                  }
                  frame #5 {
                    n495 = case shown="True" w1234 {
                      tunnel: w1235 -> [_ w1236]
                      frame False {
                      }
                      frame True {
                        n496 = while {
                          tunnel: w1236 -> [w1240]
                          stop <- w1237 continue-if-true
                          n497 = Wait Until Next ms Multiple(millisecond multiple=u32 500) -> ()  [unwired: 1 out]
                          n498 = call "GetTemperature.vi"() -> ("status"=w1238:T17, "temperature"=→"Curent Temp":i32)  [unwired: 4 in, 2 out]
                          n499 = Not Equal?(x=w1240, y=w1238) -> (x != y?=w1237:bool)
                        }
                      }
                    }
                  }
                }
              }
            }
            n500 = for {
              N: 1023 -> [_]
              tunnel: [w1210] -> w1201 mode=indexing
              i -> [w1212]
              n501 = Add(x=1, y=w1212) -> (x+y=w1210:i32)
            }
            n502 = stacked-sequence {
              seq-local: [w1243 _ _] -> [_ w1248 _]
              tunnel: TRUE -> [w1242 _ _]
              tunnel: w1204 -> [_ _ w1257]
              tunnel: w1201 -> [_ _ w1255]
              frame #0 {
                n503 = case shown="True" w1242 {
                  tunnel: [FALSE w1247] -> w1243
                  frame False {
                  }
                  frame True {
                    w1245 = 20002  # DRV_SUCCESS
                    n504 = call "StartAcquisition.vi"() -> ("DLL error code"=w1246:u32)  [unwired: 2 in, 1 out]
                    "Start Aquisition return code" <- w1246
                    n505 = Equal?(x=w1245, y=w1246) -> (x = y?=w1247:bool)
                  }
                }
              }
              frame #1 {
                n506 = case shown="True" w1248 {
                  frame False {
                  }
                  frame True {
                    n507 = while {
                      stop <- w1251 continue-if-true
                      w1250 = u16 72  # DRV ACQUIRING
                      n508 = call "GetStatus.vi"() -> ("status"=w1249:T17)  [unwired: 3 in, 2 out]
                      n509 = Wait Until Next ms Multiple(millisecond multiple=u32 50) -> ()  [unwired: 1 out]
                      n510 = property on="Get status return code" class="DigNum (strict)"("Value"=w1249) -> ()  [unwired: 2 in, 2 out]
                      n511 = Equal?(x=w1249, y=w1250) -> (x = y?=w1251:bool)
                    }
                  }
                }
              }
              frame #2 {
                n512 = call "GetAcquiredData.vi"("size"=w1257) -> ("DLL error code"=→"get aquired data return code":u32, "array"=w1254:i32[])  [unwired: 2 in, 1 out]
                n513 = Bundle(w1255, "array"=w1254) -> (→"?":cluster{i32[], "array":i32[]})  [unwired: 1 in]
                "T reached?" <- TRUE ("T reached?")
              }
            }
          }
          frame True {
            n514 = property on="T reached?" class="Bool (strict)"("Value"=FALSE ("T reached?")) -> ()  [unwired: 2 in, 2 out]
            n515 = stacked-sequence {
              frame #0 {
                n516 = call "CoolerOFF.vi"() -> ("DLL error code"=→"Cooler Off return code":u32)  [unwired: 2 in, 1 out]
              }
              frame #1 {
                n517 = while {
                  stop <- w1282 continue-if-true
                  n518 = call "GetTemperature.vi"() -> ("temperature"=w1280:i32)  [unwired: 4 in, 3 out]
                  n519 = property on="Curent Temp" class="DigNum (strict)"("Value"=w1280) -> ()  [unwired: 2 in, 2 out]
                  n520 = Less?(x=w1280, y=i16 0) -> (x < y?=w1282:bool)
                  n521 = Wait Until Next ms Multiple(millisecond multiple=u32 500) -> ()  [unwired: 1 out]
                }
              }
              frame #2 {
                n522 = call "ShutDown.vi"() -> ()  [unwired: 2 in, 2 out]
                "Shut down sequence run?" <- TRUE ("Shut down complete?")
              }
            }
          }
        }
      }
    }
    n523 = Equal To 0?(x=w23) -> (x = 0?=w34:bool)
    n524 = case shown="False" w34 {
      tunnel: w35 -> [w54 w80]
      tunnel: [w53 w78] -> w27
      tunnel: [w48 w72] -> w33
      tunnel: [w49 w73] -> w21
      tunnel: [w51 w79] -> w6
      tunnel: [w47 w71] -> w25
      tunnel: [w50 w74] -> w26
      frame False {
        n525 = call "IV getcellstatus.vi"() -> ("devcellstatus out"=w64:i32)  [unwired: 9 in, 2 out]
        n526 = call "Bitget 8-bits test.vi"("x"=w64) -> ("c"=w60:dbl, "e"=w62:dbl, "f"=w61:dbl, "h"=w63:dbl)  [unwired: 19 in, 4 out]
        n527 = Greater?(x=w60, y=0.0) -> (0:w66:bool)
        n528 = Greater?(x=w62, y=0.0) -> (0:w67:bool)
        n529 = Greater?(x=w61, y=0.0) -> (0:w68:bool)
        n530 = Greater?(x=w63, y=0.0) -> (0:w46:bool)
        n531 = And(x=w64, y=256) -> (x .and. y?=w65:i32)
        n532 = Equal?(x=w65, y=256) -> (x = y?=w69:bool)
        n533 = Bundle By Name(cluster=w54, "I overload"=w66, "Aninput1 overload"=w67, "E overload"=w68, "Cell of button pressed"=w46, "Cell on"=w69) -> (w53:T10)
        n534 = Unbundle By Name(w53) -> ("I overload"=w51:bool, "Aninput1 overload"=w50:bool, "E overload"=w49:bool, "Cell of button pressed"=w48:bool, "Cell on"=w47:bool)
      }
      frame True {
        w70 = FALSE
        # "After closing the driver reset the indicators"
        n535 = property class="XYGraph (strict)"("Value"=cluster{dbl[], dbl[]} {[], []} ("XY Graph")) -> ()  [unwired: 2 in, 2 out]
        n536 = property on="Potentiostat Status" class="Str"("Value"="" ("Device Status indicator")) -> ()  [unwired: 2 in, 2 out]
        n537 = property on="Device serial number" class="Str"("Value"="" ("Device serial number")) -> ()  [unwired: 2 in, 2 out]
        n538 = Bundle By Name(cluster=w80, "I overload"=w70, "Aninput1 overload"=w70, "E overload"=w70, "Cell of button pressed"=w70, "Cell on"=w70) -> (w78:T10)
        n539 = Unbundle By Name(w78) -> ("I overload"=w79:bool, "Aninput1 overload"=w74:bool, "E overload"=w73:bool, "Cell of button pressed"=w72:bool, "Cell on"=w71:bool)
      }
    }
    "I_overload" <- w6
    "Aninput1_overload" <- w26
    "E_overload" <- w21
    "cell-off button pressed" <- w33
    "cell on" <- w25
    n540 = Unbundle By Name(w35) -> ("Current"=→"current":dbl, "Serial No"=→"Device serial number":string, "Status"=→"Potentiostat Status":string)
    n541 = Or(x=w28, y=w40) -> (x .or. y?=w39:bool)
    n542 = Or(x=w6, y=w21) -> (x .or. y?=w20:bool)
    n543 = case shown="False" w20 {
      tunnel: w7 -> [w43 w44]
      tunnel: [w43 w44] -> w22
      frame False {
      }
      frame True {
        n544 = disable-structure shown="Disabled" {
          disable-tunnel: [State."Exit" ("f") _] -> _
          frame Disabled {
            n545 = call "Display Message to User"() -> ()  [unwired: 10 in, 2 out]
          }
          frame Enabled {
          }
        }
      }
    }
  }
